vi "CRT Controller.vi"() -> ()   [LabVIEW 2016]
uses:
  HPTDC Driver Library Folder/Library files/Typedefs/TDCManager.ctl
  HPTDC Driver Library Folder/Library files/Typedefs/TDCHit.ctl
  VIs/Typedefs/Coincidence single histogram.ctl
  VIs/Typedefs/HitChart.ctl
  VIs/Typedefs/ROB display info.ctl
  <vilib>/addons/h5labview2/base/hid_t.ctl
  VIs/Typedefs/Hit chart cluster refnum.ctl
  <vilib>/Platform/TimedLoop/XDataNode/timing_clust.ctl
  <vilib>/Platform/TimedLoop/XDataNode/nitl_modes.ctl
  <vilib>/Platform/TimedLoop/XDataNode/wakeup.ctl
  HPTDC Driver Library Folder/Library files/Typedefs/TDCManagerRefnum.ctl
  VIs/Global Variables/Global AllowRead.vi
  VIs/Global Variables/AllowTDCHitsRead.vi
  VIs/Global Variables/AllowTDCFastRead.vi
  VIs/Global Variables/take CRT data.vi
  VIs/Global Variables/Master Ready For Data.vi
  VIs/Global Variables/Coincidence hunt limit.vi
  VIs/Global Variables/Program load indicators.vi
  VIs/Global Variables/AllowUserMessages.vi
  VIs/Global Variables/Coincidence Windows.vi
  VIs/Global Variables/System info.vi
  <vilib>/Instr/_visa.llb/VISA Configure Serial Port (Instr).vi
  <vilib>/platform/TimedLoop/XDataNode/XDataNode.xnode
  HPTDC Driver Library Folder/HPTDC Driver Library.lvlib
  <vilib>/Platform/TimedLoop/XDataNode/XDNodeRunTimeDep.lvlib
  <vilib>/addons/h5labview2/file/H5F.lvlib
  C:/Users/CRT Controller/CRTC Labview Application/Source/HPTDC Driver Library Folder/Library files/hptdc_net4_3.7.0_x64.dll
  HPTDC Driver Library Folder/Library files/hptdc_net4_3.7.0_x64.dll
panel:
  out "charactirzator refnum":refnum<vi>
  out "TDC Command Queue":string[](array[string])
  in  "Tab Control":T1(tab)
  in  "Hit rate save granularity in minutes":i32=1 min=1 step=1
  in  "GPS information save granularity in minutes":i32=1 min=1 step=1
  out "TDCRead":dbl(knob) scale=0.0..3300.0
  in  "Open coincrate":bool
  in  "Open trigrate":bool
  in  "Open EventDisplay":bool
  out "Run initiated at":timestamp
  out "Run ID":i32
  in  "Start Run":bool
  in  "ROB information save granularity in minutes":i32=15 min=1 step=1
  out "~Reads/s":u64
  in  "Planar coincidence window":i32=5 min=1 step=1 format="±%d ns"
  in  "Coincidence grouping window":i32=10 format="%d ns"
  out "Coincidences analysis overload":bool
  out "Coinchunt overflow":bool caption="Coincidence hunt overload"
  out "TDCRead overflow":bool caption="TDC readout overload"
  out "Sorter overflow":bool caption="Sorter overload"
  out "Coincidencehunt limit":dbl(knob) scale=0.0..900.0
  in  "Disable rail monitor":bool
  in  "Disable 15":bool
  in  "Enable 15":bool
  in  "Disable auto latch reset":bool
  in  "Verbosity":u8
  in  "Set Debug Verbosity":bool
  in  "Overvoltage":sgl=3.0 min=0 max=100 step=0.01 format="%#_4g V"
  in  "Set MPPCovervoltage":bool
  in  "Rep trigthres":bool
  in  "ROB hard reset":bool
  in  "disable amp":bool
  in  "Enable amp":bool caption="Enable"
  in  "Enable usermessages":bool=TRUE
  in  "Reset latch":bool
  in  "disable +-5V":bool
  in  "Enable +-5":bool
  in  "Disable 3.3":bool
  in  "Enable 3.3":bool
  in  "Voltage ref":u16(ring) items=["Default (internal)", "External"]
  in  "Continuous test charge":bool
  in  "Rep Temp":bool
  in  "Hard-set value":bool
  in  "VTrig mV":sgl min=0 max=1000 step=1 format="%#_2g mV"
  in  "Disable auto-VBias":bool
  in  "Bias voltage":sgl min=0 max=100 step=0.01 format="%#_4g V"
  in  "Set MPPC Bias":bool
  in  "VTrig percent":sgl min=0 max=100 step=0.1 format="%#_4g %"
  in  "Set VTrig":bool
  in  "Board selector":u16(ring) items=["0", "1", "2", "3", "4", "5", "6", "7", "8", "9", "10", "11", "12", "13", "14", "15", "All boards"]
  in  "go to standby":bool
  in  "Go to ready":bool
  in  "go to running":bool
  in  "Rep voltages":bool
  in  "Rep status":bool
  in  "Rep disclatch":bool
  in  "Remove MPPC":bool
  in  "Insert test charge":bool
  in  "Set voltage reference":bool
  in  "Echo":bool
  out "ROB Info cluster":T3={"ROB Info-display"={"ID:"=0, "State:"="UNKNOWN", "Voltages"=-1, "Temp:"=-1.0, "Latch count:"=-1, "VRef:"=enum."Unknown", "Trigthres:"=-1, "MPPC EN"=FALSE, "Test charge"=FALSE, "Responding"=FALSE, "Last update"=timestamp(0 s since 1904-01-01)}, "ROB Info-display 2"={"ID:"=1, "State:"="UNKNOWN", "Voltages"=-1, "Temp:"=-1.0, "Latch count:"=-1, "VRef:"=enum."Unknown", "Trigthres:"=-1, "MPPC EN"=FALSE, "Test charge"=FALSE, "Responding"=FALSE, "Last update"=timestamp(0 s since 1904-01-01)}, "ROB Info-display 3"={"ID:"=2, "State:"="UNKNOWN", "Voltages"=-1, "Temp:"=-1.0, "Latch count:"=-1, "VRef:"=enum."Unknown", "Trigthres:"=-1, "MPPC EN"=FALSE, "Test charge"=FALSE, "Responding"=FALSE, "Last update"=timestamp(0 s since 1904-01-01)}, "ROB Info-display 4"={"ID:"=3, "State:"="UNKNOWN", "Voltages"=-1, "Temp:"=-1.0, "Latch count:"=-1, "VRef:"=enum."Unknown", "Trigthres:"=-1, "MPPC EN"=FALSE, "Test charge"=FALSE, "Responding"=FALSE, "Last update"=timestamp(0 s since 1904-01-01)}, "ROB Info-display 5"={"ID:"=4, "State:"="UNKNOWN", "Voltages"=-1, "Temp:"=-1.0, "Latch count:"=-1, "VRef:"=enum."Unknown", "Trigthres:"=-1, "MPPC EN"=FALSE, "Test charge"=FALSE, "Responding"=FALSE, "Last update"=timestamp(0 s since 1904-01-01)}, "ROB Info-display 6"={"ID:"=5, "State:"="UNKNOWN", "Voltages"=-1, "Temp:"=-1.0, "Latch count:"=-1, "VRef:"=enum."Unknown", "Trigthres:"=-1, "MPPC EN"=FALSE, "Test charge"=FALSE, "Responding"=FALSE, "Last update"=timestamp(0 s since 1904-01-01)}, "ROB Info-display 7"={"ID:"=6, "State:"="UNKNOWN", "Voltages"=-1, "Temp:"=-1.0, "Latch count:"=-1, "VRef:"=enum."Unknown", "Trigthres:"=-1, "MPPC EN"=FALSE, "Test charge"=FALSE, "Responding"=FALSE, "Last update"=timestamp(0 s since 1904-01-01)}, "ROB Info-display 8"={"ID:"=7, "State:"="UNKNOWN", "Voltages"=-1, "Temp:"=-1.0, "Latch count:"=-1, "VRef:"=enum."Unknown", "Trigthres:"=-1, "MPPC EN"=FALSE, "Test charge"=FALSE, "Responding"=FALSE, "Last update"=timestamp(0 s since 1904-01-01)}, "ROB Info-display 9"={"ID:"=8, "State:"="UNKNOWN", "Voltages"=-1, "Temp:"=-1.0, "Latch count:"=-1, "VRef:"=enum."Unknown", "Trigthres:"=-1, "MPPC EN"=FALSE, "Test charge"=FALSE, "Responding"=FALSE, "Last update"=timestamp(0 s since 1904-01-01)}, "ROB Info-display 10"={"ID:"=9, "State:"="UNKNOWN", "Voltages"=-1, "Temp:"=-1.0, "Latch count:"=-1, "VRef:"=enum."Unknown", "Trigthres:"=-1, "MPPC EN"=FALSE, "Test charge"=FALSE, "Responding"=FALSE, "Last update"=timestamp(0 s since 1904-01-01)}, "ROB Info-display 11"={"ID:"=10, "State:"="UNKNOWN", "Voltages"=-1, "Temp:"=-1.0, "Latch count:"=-1, "VRef:"=enum."Unknown", "Trigthres:"=-1, "MPPC EN"=FALSE, "Test charge"=FALSE, "Responding"=FALSE, "Last update"=timestamp(0 s since 1904-01-01)}, "ROB Info-display 12"={"ID:"=11, "State:"="UNKNOWN", "Voltages"=-1, "Temp:"=-1.0, "Latch count:"=-1, "VRef:"=enum."Unknown", "Trigthres:"=-1, "MPPC EN"=FALSE, "Test charge"=FALSE, "Responding"=FALSE, "Last update"=timestamp(0 s since 1904-01-01)}, "ROB Info-display 13"={"ID:"=12, "State:"="UNKNOWN", "Voltages"=-1, "Temp:"=-1.0, "Latch count:"=-1, "VRef:"=enum."Unknown", "Trigthres:"=-1, "MPPC EN"=FALSE, "Test charge"=FALSE, "Responding"=FALSE, "Last update"=timestamp(0 s since 1904-01-01)}, "ROB Info-display 14"={"ID:"=13, "State:"="UNKNOWN", "Voltages"=-1, "Temp:"=-1.0, "Latch count:"=-1, "VRef:"=enum."Unknown", "Trigthres:"=-1, "MPPC EN"=FALSE, "Test charge"=FALSE, "Responding"=FALSE, "Last update"=timestamp(0 s since 1904-01-01)}, "ROB Info-display 15"={"ID:"=14, "State:"="UNKNOWN", "Voltages"=-1, "Temp:"=-1.0, "Latch count:"=-1, "VRef:"=enum."Unknown", "Trigthres:"=-1, "MPPC EN"=FALSE, "Test charge"=FALSE, "Responding"=FALSE, "Last update"=timestamp(0 s since 1904-01-01)}, "ROB Info-display 16"={"ID:"=15, "State:"="UNKNOWN", "Voltages"=-1, "Temp:"=-1.0, "Latch count:"=-1, "VRef:"=enum."Unknown", "Trigthres:"=-1, "MPPC EN"=FALSE, "Test charge"=FALSE, "Responding"=FALSE, "Last update"=timestamp(0 s since 1904-01-01)}} {"ROB Info-display 16"."Last update" format="%<%X>T"; "ROB Info-display 16"."Trigthres:" format="%.0fmV"; "ROB Info-display 16"."Temp:" format="%.2f C"; "ROB Info-display 15"."Last update" format="%<%X>T"; "ROB Info-display 15"."Trigthres:" format="%.0fmV"; "ROB Info-display 15"."Temp:" format="%.2f C"; "ROB Info-display 14"."Last update" format="%<%X>T"; "ROB Info-display 14"."Trigthres:" format="%.0fmV"; "ROB Info-display 14"."Temp:" format="%.2f C"; "ROB Info-display 13"."Last update" format="%<%X>T"; "ROB Info-display 13"."Trigthres:" format="%.0fmV"; "ROB Info-display 13"."Temp:" format="%.2f C"; "ROB Info-display 12"."Last update" format="%<%X>T"; "ROB Info-display 12"."Trigthres:" format="%.0fmV"; "ROB Info-display 12"."Temp:" format="%.2f C"; "ROB Info-display 11"."Last update" format="%<%X>T"; "ROB Info-display 11"."Trigthres:" format="%.0fmV"; "ROB Info-display 11"."Temp:" format="%.2f C"; "ROB Info-display 10"."Last update" format="%<%X>T"; "ROB Info-display 10"."Trigthres:" format="%.0fmV"; "ROB Info-display 10"."Temp:" format="%.2f C"; "ROB Info-display 9"."Last update" format="%<%X>T"; "ROB Info-display 9"."Trigthres:" format="%.0fmV"; "ROB Info-display 9"."Temp:" format="%.2f C"; "ROB Info-display 8"."Last update" format="%<%X>T"; "ROB Info-display 8"."Trigthres:" format="%.0fmV"; "ROB Info-display 8"."Temp:" format="%.2f C"; "ROB Info-display 7"."Last update" format="%<%X>T"; "ROB Info-display 7"."Trigthres:" format="%.0fmV"; "ROB Info-display 7"."Temp:" format="%.2f C"; "ROB Info-display 6"."Last update" format="%<%X>T"; "ROB Info-display 6"."Trigthres:" format="%.0fmV"; "ROB Info-display 6"."Temp:" format="%.2f C"; "ROB Info-display 5"."Last update" format="%<%X>T"; "ROB Info-display 5"."Trigthres:" format="%.0fmV"; "ROB Info-display 5"."Temp:" format="%.2f C"; "ROB Info-display 4"."Last update" format="%<%X>T"; "ROB Info-display 4"."Trigthres:" format="%.0fmV"; "ROB Info-display 4"."Temp:" format="%.2f C"; "ROB Info-display 3"."Last update" format="%<%X>T"; "ROB Info-display 3"."Trigthres:" format="%.0fmV"; "ROB Info-display 3"."Temp:" format="%.2f C"; "ROB Info-display 2"."Last update" format="%<%X>T"; "ROB Info-display 2"."Trigthres:" format="%.0fmV"; "ROB Info-display 2"."Temp:" format="%.2f C"; "ROB Info-display"."Last update" format="%<%X>T"; "ROB Info-display"."Trigthres:" format="%.0fmV"; "ROB Info-display"."Temp:" format="%.2f C"}
  in  "enable autoread":bool
  in  "enable rail monitor":bool
  in  "Fast read":bool caption="Only register amount of hits, \nnot time or channel. Supports reading \nout at the maximum TDC speed."
  out "Status":u16(ring) items=["Uninitialized", "Not configured", "Configured", "Running", "Paused", "Shutdown"]
  in  "Continue tdc":bool
  in  "Pause tdc":bool
  in  "Stop tdc":bool
  in  "Start tdc":bool
  in  "Read Cfg Again":bool
  in  "Reconfigure":bool
  in  "Read config string":bool
  in  "TDC Config string":string="FallingEnable 1"
  out "Set Parameter Names":string[](array[string])
  in  "Get set param names":bool
  in  "TDC Configuration filepath":string="C:\\Users\\CRT Controller\\CRTC Labview Application\\Source\\global.cfg"
  out "Init success":bool
  out "Histograms cluster":T5 {"Cluster 33"."S:" format="%_3f"; "Cluster 32"."S:" format="%_3f"; "Cluster 31"."S:" format="%_3f"; "Cluster 30"."S:" format="%_3f"; "Cluster 29"."S:" format="%_3f"; "Cluster 28"."S:" format="%_3f"; "Cluster 27"."S:" format="%_3f"; "Cluster 26"."S:" format="%_3f"; "Cluster 25"."S:" format="%_3f"; "Cluster 24"."S:" format="%_3f"; "Cluster 23"."S:" format="%_3f"; "Cluster 22"."S:" format="%_3f"; "Cluster 21"."S:" format="%_3f"; "Cluster 20"."S:" format="%_3f"; "Cluster 19"."S:" format="%_3f"; "Cluster 18"."S:" format="%_3f"; "Cluster 17"."S:" format="%_3f"; "Cluster 16"."S:" format="%_3f"; "Cluster 15"."S:" format="%_3f"; "Cluster 14"."S:" format="%_3f"; "Cluster 13"."S:" format="%_3f"; "Cluster 12"."S:" format="%_3f"; "Cluster 11"."S:" format="%_3f"; "Cluster 10"."S:" format="%_3f"; "Cluster 9"."S:" format="%_3f"; "Cluster 8"."S:" format="%_3f"; "Cluster 7"."S:" format="%_3f"; "Cluster 6"."S:" format="%_3f"; "Cluster 5"."S:" format="%_3f"; "Cluster 4"."S:" format="%_3f"; "Cluster 3"."S:" format="%_3f"; "Cluster 2"."S:" format="%_3f"}
  in  "Histogram select":T6(ring)
  in  "MaxHistItems":i32=1000 caption="Number of elements"
  in  "SetMaxHistItems":bool
  in  "charts tab":enum32{"Top layer", "Bottom layer"}(tab)
  out "Top layer hit charts":T8 {"Waveform Chart 8"."ID" format="ch %d"; "Waveform Chart 7"."ID" format="ch %d"; "Waveform Chart 6"."ID" format="ch %d"; "Waveform Chart 5"."ID" format="ch %d"; "Waveform Chart 4"."ID" format="ch %d"; "Waveform Chart 3"."ID" format="ch %d"; "Waveform Chart 2"."ID" format="ch %d"; "Waveform Chart"."ID" format="ch %d"}
  out "Bottom layer hit charts":T8 {"Waveform Chart 8"."ID" format="ch %d"; "Waveform Chart 7"."ID" format="ch %d"; "Waveform Chart 6"."ID" format="ch %d"; "Waveform Chart 5"."ID" format="ch %d"; "Waveform Chart 4"."ID" format="ch %d"; "Waveform Chart 3"."ID" format="ch %d"; "Waveform Chart 2"."ID" format="ch %d"; "Waveform Chart"."ID" format="ch %d"}
  in  "Resolution(seconds)":dbl=5.0 min=0.1 step=1.0
  in  "Set chart res":bool
  in  "Clear charts":bool
  out "Coinc stats time":i32 caption="Seconds of coincidence statistics:"
  out "Coinc stats table":string[][](table) caption="Statistics of the latest coincidences"
  in  "GPS CMD Send Button":bool
  in  "GPS command input":string
  in  "Baud rate GPS":u32=38400 caption="Baud rate"
  in  "GPS serial port":refnum<visa-resource-name>="COM7"
  in  "Open GPS Port":bool caption="Open ROB Port"
  in  "Open Master Port":bool
  in  "Baud rate sniffer":u32=9600 caption="Baud rate"
  in  "Sniffer serial port":refnum<visa-resource-name>
  in  "Open Sniffer Port":bool
  in  "Baud rate ROB":u32=9600 caption="Baud rate"
  in  "ROB serial port":refnum<visa-resource-name>
  in  "Open ROB Port":bool
  in  "Baud rate master":u32=115200 caption="Baud rate"
  in  "Master serial port":refnum<visa-resource-name>="COM3"
  out "Master Serial Input Data":string
  out "Sniffer Serial Input Data":string
  out "ROB Serial Input Data":string
  out "GPS serial input data":string
  out "Initiate finished":bool
  out "Programmatic set trigthres":bool
  in  "Data recording root path":path=path "D:/Data/2018"
  in  "run counter path":path=path "C:/Users/CRT Controller/CRTC Labview Application/Source/Configurations etc/Run counter.txt"
  out "Programmatic rep disclatch":bool
  out "Programmatic rep temp":bool
  out "Programmatic rep stat":bool
  out "Programmatic rep volts":bool
  out "Command Queue":string[](array[string])
  out "StopNotifier":refnum<notifier>
  out "Sniffer serial port":refnum<visa-resource-name>
  out "ROB serial port":refnum<visa-resource-name>
  out "Master serial port":refnum<visa-resource-name>
  out "TDCHitsQueue":refnum<queue>
  in  "TDCManager":T9
  out "Master data":u8[][](array[numeric])
  out "Sorter Refnum":refnum<vi>
  out "TDCRead Refnum":refnum<vi>
  out "TDCFastRead Refnum":refnum<vi>
  out "MasterSerial Refnum":refnum<vi>
  out "SnifferSerial Refnum":refnum<vi>
  out "ROBSerial Refnum":refnum<vi>
  out "Daily datafile reference":T10 format="%.0x"
  out "Master command sender refnum":refnum<vi>
  out "Added time":u64
  out "Coinchunt Lim":i32
  out "MasterCmdQueue":refnum<queue>
  out "error out":errorcluster
  out "TDCStart time":timestamp
  out "Event display Refnum":refnum<vi>
  out "Current day":i32
  out "Trig chara refnum":refnum<vi>
  out "GPS serial port":refnum<visa-resource-name>
  out "GPSSerial Refnum":refnum<vi>
  out "GpsDataQueue":refnum<queue>
  out "hit charts refnum cluster":T12
  in  "stop":bool
  # "Debug things. No need to touch this in normal operation..."
  # "Rail monitor"
  # "15V"
  # "3.3V"
  # "+-5V"
  # "Amplifier"
  # "This table shows the total amount of registered coincidences over the last 10000 seconds or so. The top coloumns indicates that, for a block of coincidences, how many were present in the top plane. The rows indicate how many were present in the bottom plane. \nSo if 1x1 has the highest number, that means it is most common for a single coincidence on the top plane and a single coincidence on the bottom plane to occur simulatenously (within the CRT-wide coincidence window).\nIt is unlikely that more than a few coincidences will occur simulatenously, but up to 10x10 has been added to the table to spot unforeseen problems."
  # "These items are internal variables used by the CRTC and \ncannot be modified or should not be modified."
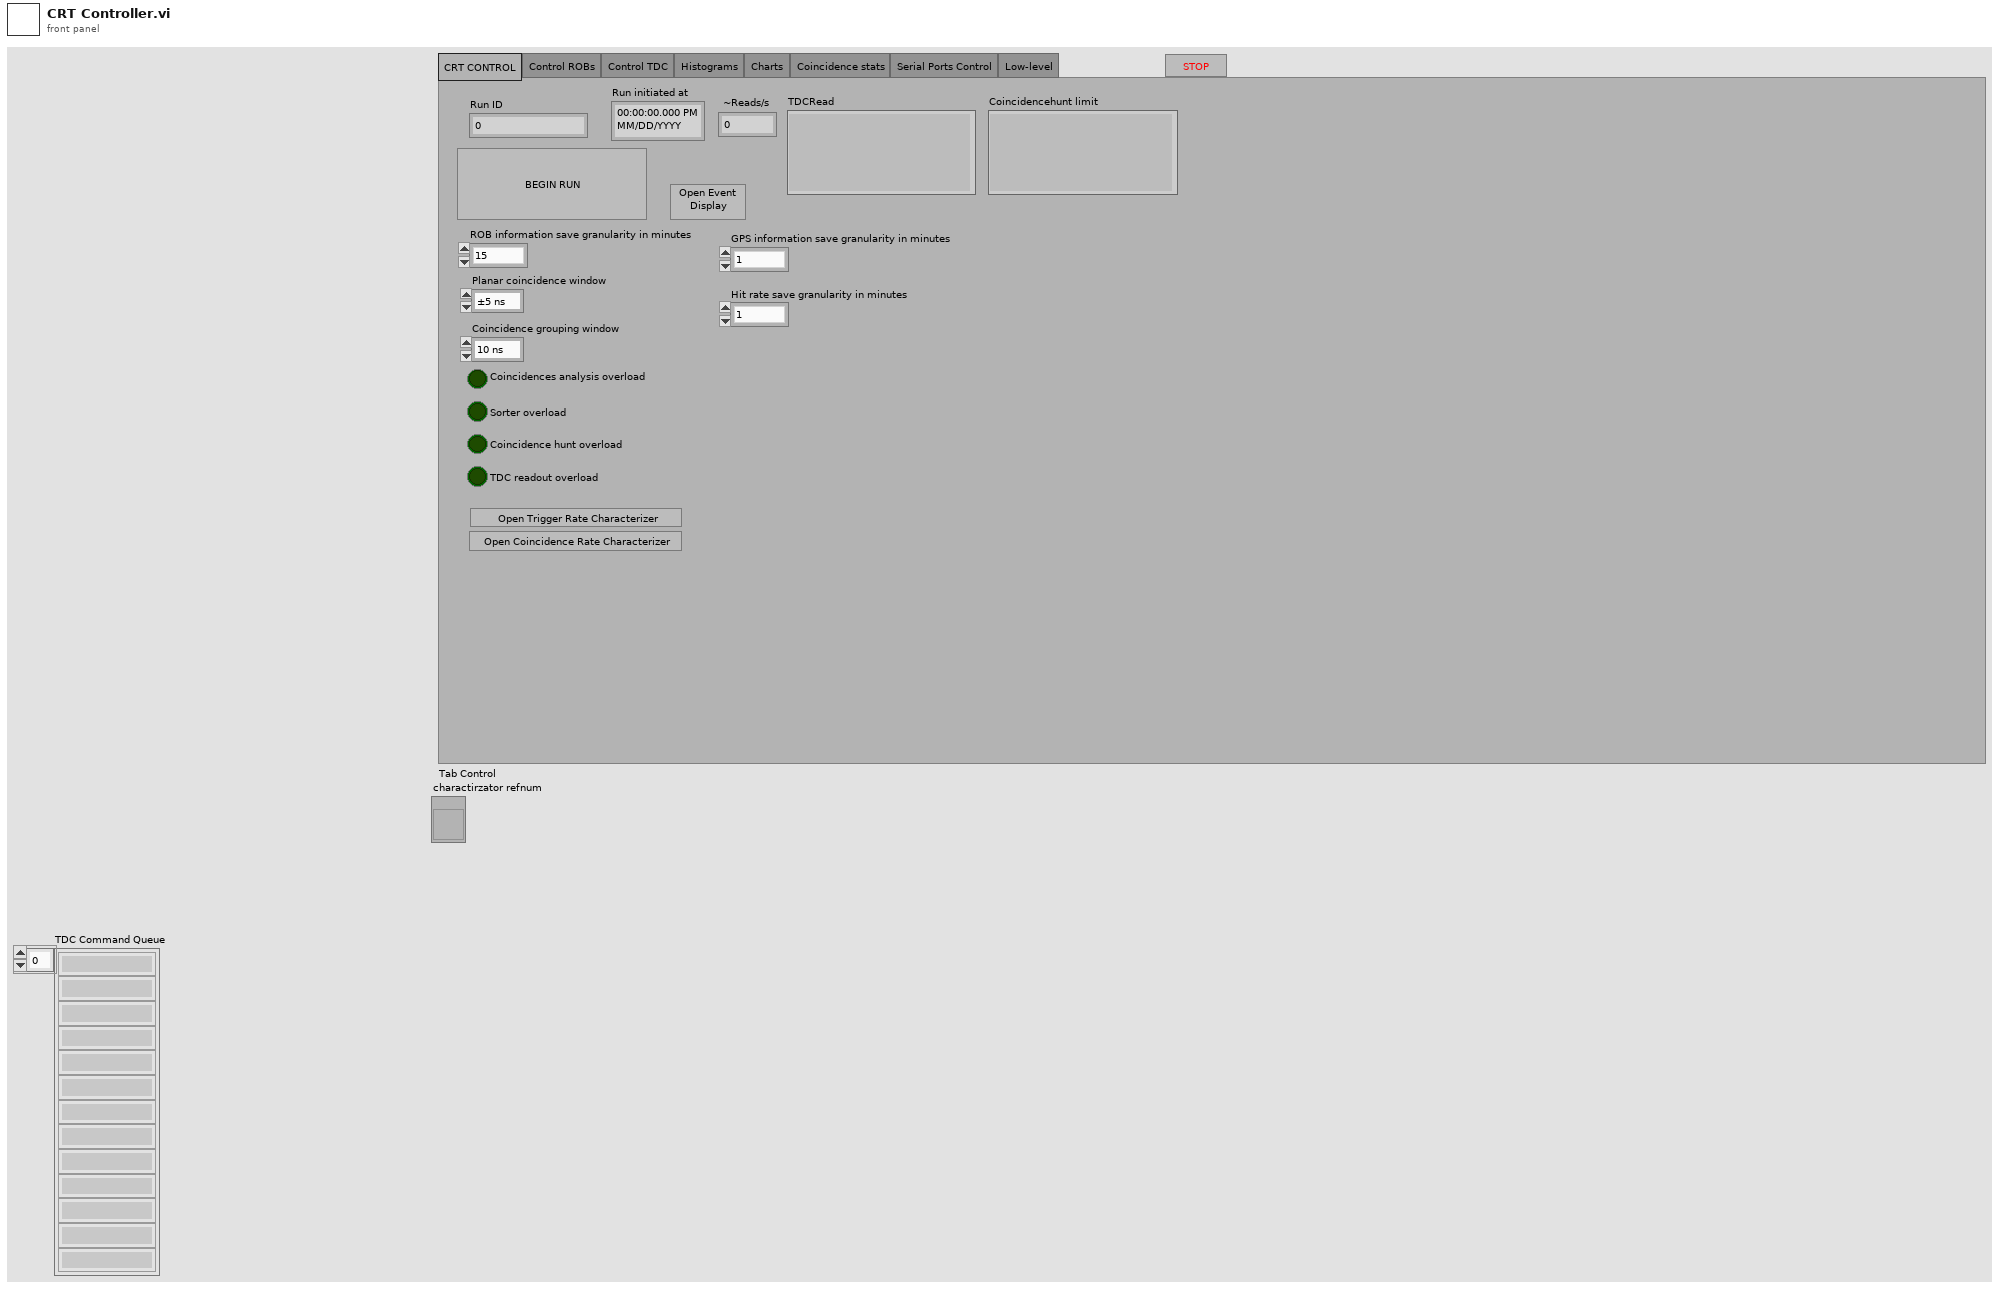
[diagram p1: front panel]
types:
  T1 = enum32{"CRT CONTROL", "Control ROBs", "Control TDC", "Histograms", "Charts", "Coincidence stats", "Serial Ports Control", "Low-level"}
  T2 = typedef "ROB display info.ctl" = cluster{"ID:":i32, "State:":string, "Voltages":i32, "Temp:":dbl, "Latch count:":i32, "VRef:":enum16{"External", "Internal", "Unknown"}, "Trigthres:":i32, "MPPC EN":bool, "Test charge":bool, "Responding":bool, "Last update":timestamp}
  T3 = cluster{"ROB Info-display":T2, "ROB Info-display 2":T2, "ROB Info-display 3":T2, "ROB Info-display 4":T2, "ROB Info-display 5":T2, "ROB Info-display 6":T2, "ROB Info-display 7":T2, "ROB Info-display 8":T2, "ROB Info-display 9":T2, "ROB Info-display 10":T2, "ROB Info-display 11":T2, "ROB Info-display 12":T2, "ROB Info-display 13":T2, "ROB Info-display 14":T2, "ROB Info-display 15":T2, "ROB Info-display 16":T2}
  T4 = typedef "Coincidence single histogram.ctl" = cluster{"Histogram Graph":cluster{"X Values":dbl[], "Histogram: h(x)":i32[]}[], "IDs":i8[], "Datapoints:":i32, "S:":dbl, "Data array":cluster{"Data":i32[], "Max index":i32, "Current index":i32, "Numofpoints":i32}}
  T5 = cluster{"Cluster 2":T4, "Cluster 3":T4, "Cluster 4":T4, "Cluster 5":T4, "Cluster 6":T4, "Cluster 7":T4, "Cluster 8":T4, "Cluster 9":T4, "Cluster 10":T4, "Cluster 11":T4, "Cluster 12":T4, "Cluster 13":T4, "Cluster 14":T4, "Cluster 15":T4, "Cluster 16":T4, "Cluster 17":T4, "Cluster 18":T4, "Cluster 19":T4, "Cluster 20":T4, "Cluster 21":T4, "Cluster 22":T4, "Cluster 23":T4, "Cluster 24":T4, "Cluster 25":T4, "Cluster 26":T4, "Cluster 27":T4, "Cluster 28":T4, "Cluster 29":T4, "Cluster 30":T4, "Cluster 31":T4, "Cluster 32":T4, "Cluster 33":T4}
  T6 = enum16{"All histograms", "0x4", "0x5", "0x6", "0x7", "1x4", "1x5", "1x6", "1x7", "2x4", "2x5", "2x6", "2x7", "3x4", "3x5", "3x6", "3x7", "8x12", "8x13", "8x14", "8x15", "9x12", "9x13", "9x14", "9x15", "10x12", "10x13", "10x14", "10x15", "11x12", "11x13", "11x14", "11x15"}
  T7 = typedef "HitChart.ctl" = cluster{"Waveform Chart":cluster{"Coincidences":dbl, "Non-coincidences":dbl, "Ratio":dbl, "Total hits":dbl}[], "Last update timestamp":timestamp, "Resolution(s)":dbl, "nondisplayed coincs":i32, "nondisplayed noncoincs":i32, "Last upd":i64, "ID":i8}
  T8 = cluster{"Waveform Chart":T7, "Waveform Chart 2":T7, "Waveform Chart 3":T7, "Waveform Chart 4":T7, "Waveform Chart 5":T7, "Waveform Chart 6":T7, "Waveform Chart 7":T7, "Waveform Chart 8":T7}
  T9 = typedef "HPTDC Driver Library.lvlib/TDCManager.ctl" = refnum<k24>
  T10 = typedef "hid_t.ctl" = i32
  T11 = typedef "Hit chart cluster refnum.ctl" = refnum<vi>
  T12 = cluster{"Hit charts top":T11, "Hit charts bottom":T11}
  T13 = cluster{"Data":string, "Port":refnum<visa-resource-name>}
  T14 = typedef "HPTDC Driver Library.lvlib/TDCHit.ctl" = cluster{"channel":u8, "time":u64, "type":u8}
  T15 = typedef "XDNodeRunTimeDep.lvlib/timing_clust.ctl" = cluster{"Expected End [f-1]":u64, "Actual End [f-1]":u64, "Finished Late? [f-1]":bool, "Expected End [i-1]":u64, "Actual End [i-1]":u64, "Finished Late? [i-1]":bool, "Expected Start [i]":u64, "Actual Start [i]":u64, "Expected Start [f]":u64, "Actual Start [f]":u64, "Source Name":string, "Structure Name":string, "Period":i64, "Deadline":i64, "Offset":i64, "Start":i64, "Priority":i32, "Timeout":i32, "Mode":T16, "Wakeup Reason":T17, "Error":errorcluster, "Source Type":string, "Secondary Source Type":string, "Global End Time":u64, "Global Start Time":u64, "Frame Duration":u64, "Iteration Duration":u64, "Assigned CPU":i32, "I/O Scan Engine Mode":u32}
  T16 = typedef "XDNodeRunTimeDep.lvlib/nitl_modes.ctl" = enum32{"No Change", "Process missed periods, maintain original phase", "Discard missed periods, maintain original phase", "Process missed periods, ignore original phase", "Discard missed periods, ignore original phase"}
  T17 = typedef "XDNodeRunTimeDep.lvlib/wakeup.ctl" = enum32{"Normal", "Aborted", "Asynchronous wakeup", "Timing source error", "Timed loop error", "Timeout"}
  T18 = enum16{"Reset", "ReadAndReset", "Read", "Add", "Init"}
  T19 = enum16{"big-endian, network order", "native, host order", "little-endian"}
  T20 = enum8{"Enabled", "Disabled", "Disabled and Grayed Out"}
  T21 = enum32{"Invalid", "Standard", "Closed", "Hidden", "Minimized", "Maximized"}
  T22 = cluster{"VTrig mV":refnum<vi>, "Top hit charts":T11, "Bottom hit charts":T11, "Board selector":refnum<vi>, "VTrig percent ":refnum<vi>, "Hard-set value":refnum<vi>, "Programmatic set trigthres":refnum<vi>}
  T23 = enum16{"insertPPS", "insertUTC", "read", "initiate"}
  T24 = cluster{"VISAResourceName in":refnum<vi>, "Input buffer refnum":refnum<vi>}
  T25 = cluster{"Master data ref":refnum<vi>, "VISAResourceName in":refnum<vi>, "Input buffer refnum":refnum<vi>}
  T26 = typedef "TDCManagerRefnum.ctl" = refnum<vi>
  T27 = cluster{"TDCManager Refnum":T26, "Unable to keep up indicator":refnum<vi>}
  T28 = cluster{"TDCManager Refnum":T26, "Queue overflow indicator":refnum<vi>, "Hit rate warning":refnum<vi>}
  T29 = typedef "Semaphore RefNum" = refnum<k1>
  T30 = cluster{"Hit charts bottom":T11, "Hit charts top":T11, "Hitrate save granularity in minutes":refnum<vi>}
  T31 = enum16{"Null", "BottomLayer", "TopAndBottom", "TopLayer"}
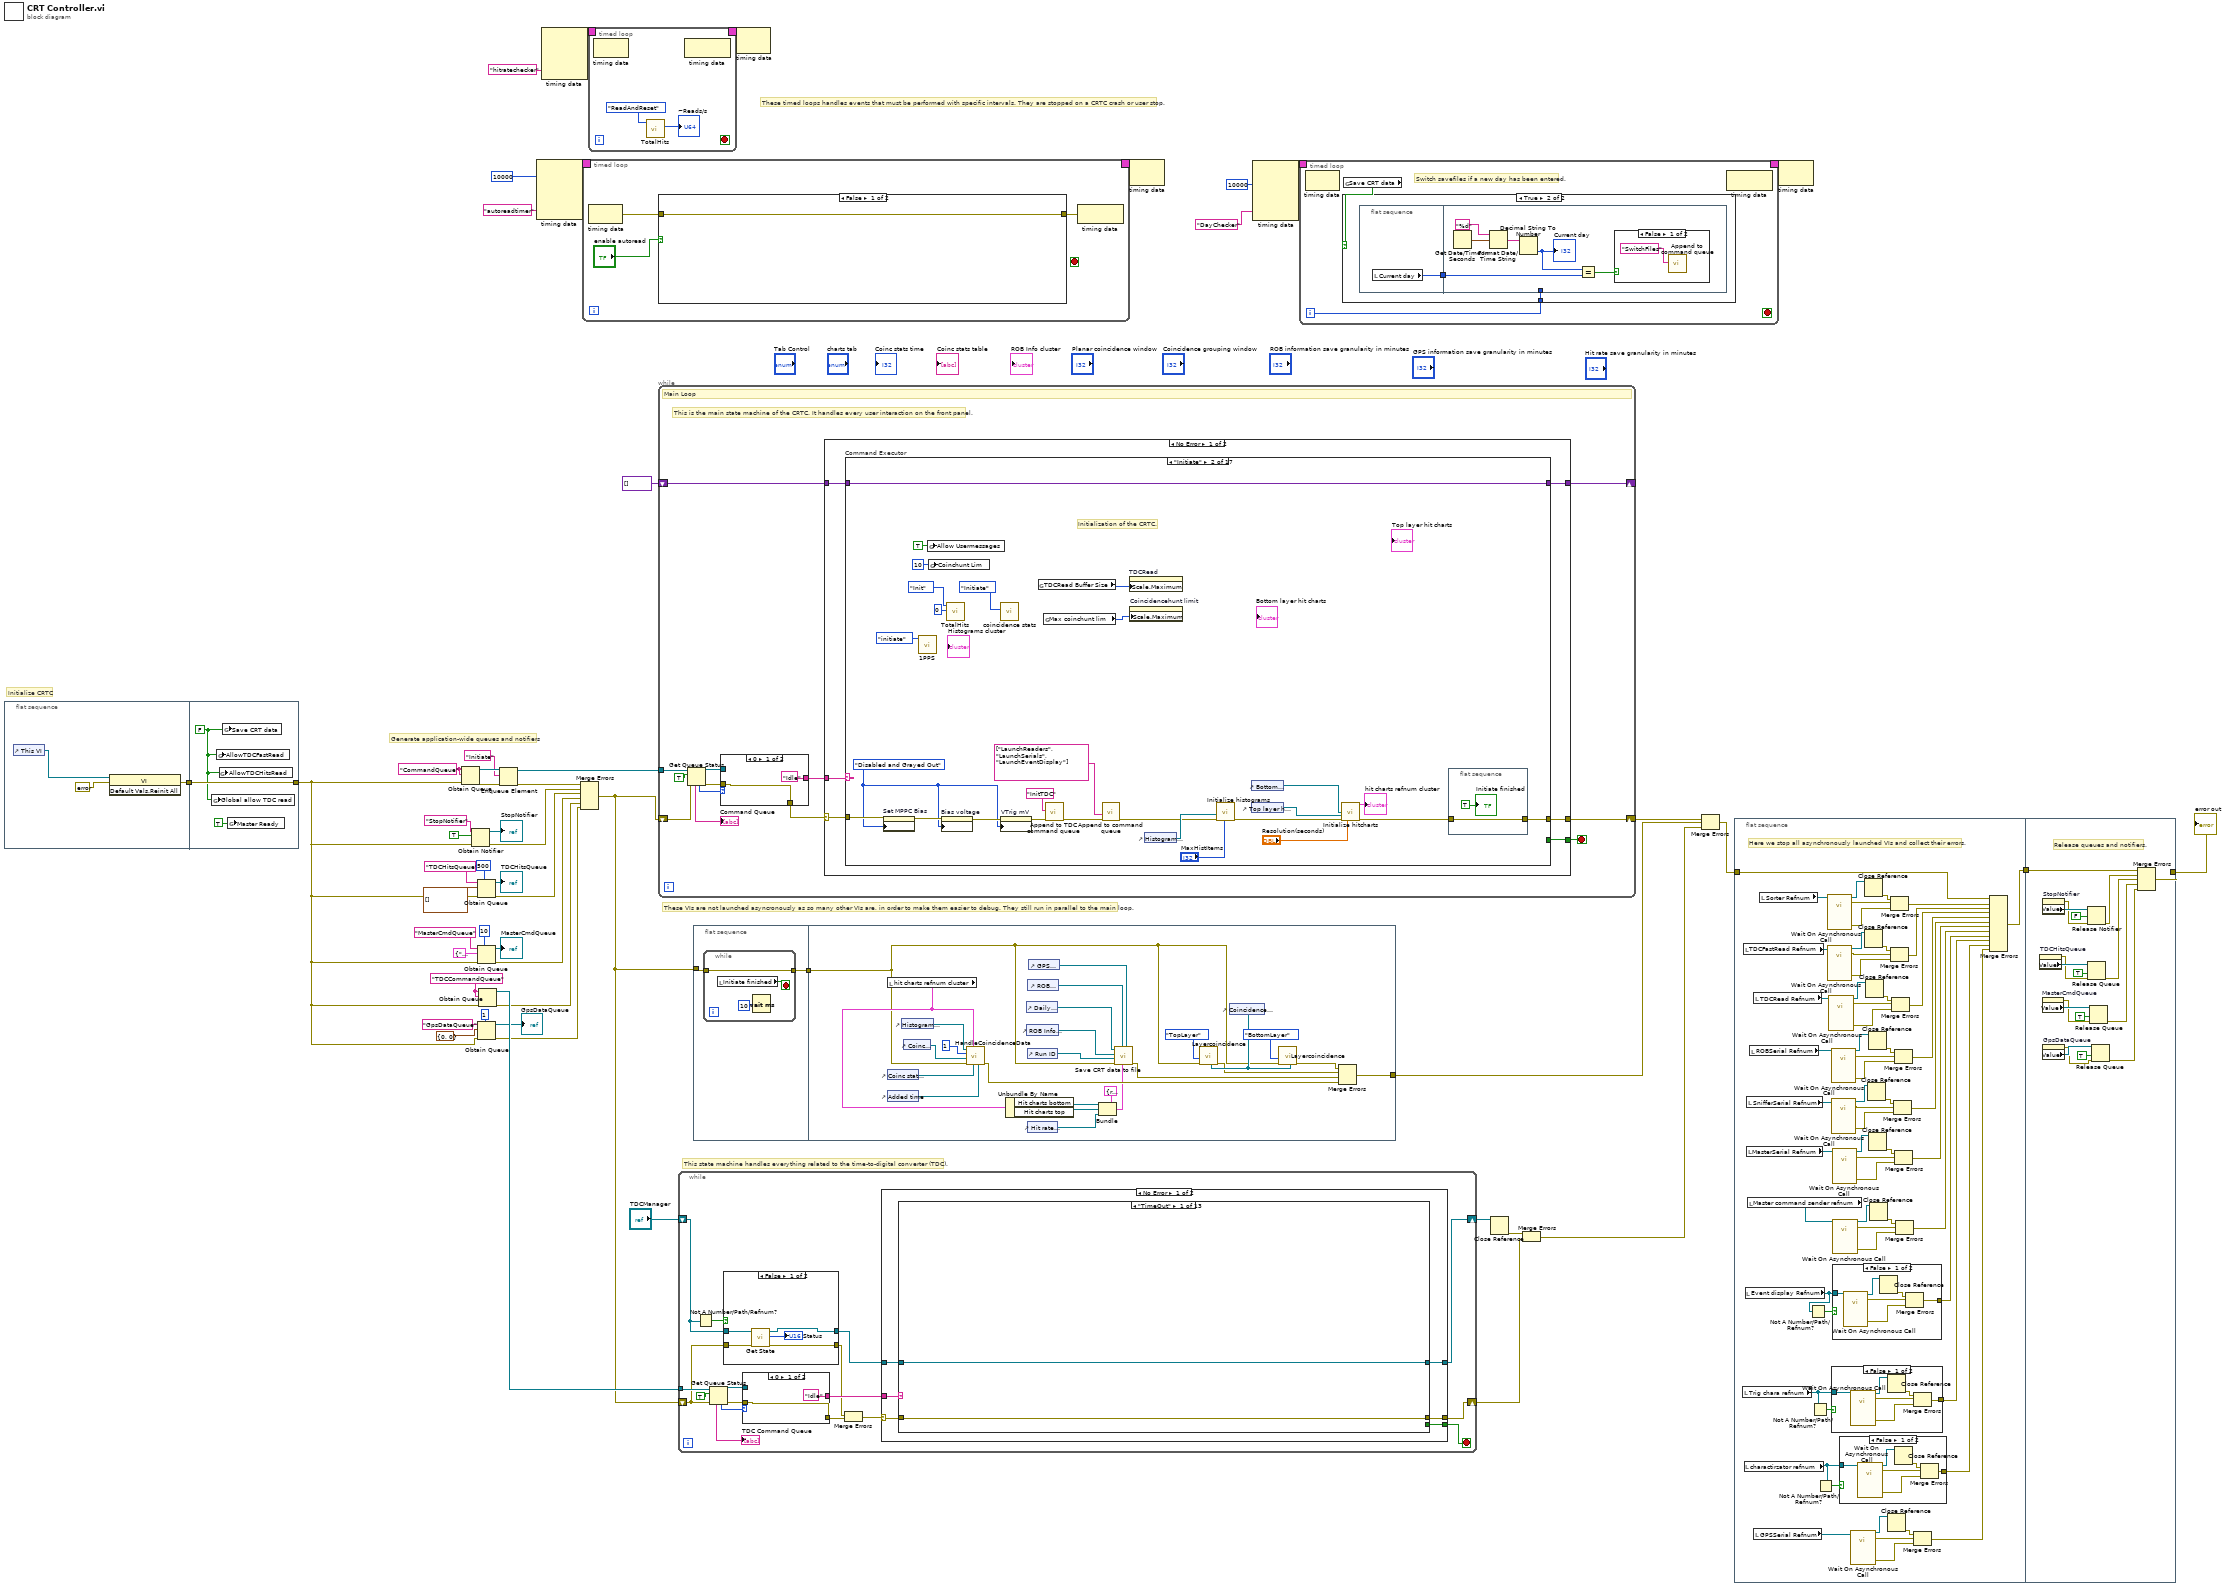
[diagram p0: block diagram]
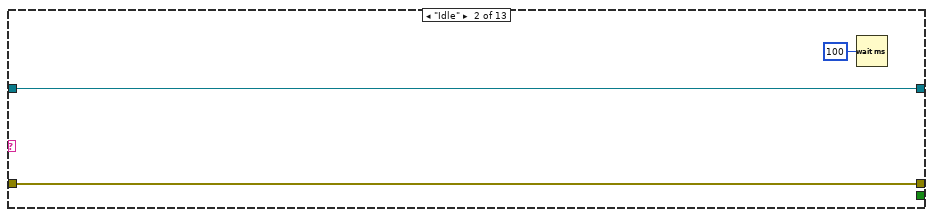
[diagram p3: hidden frame]
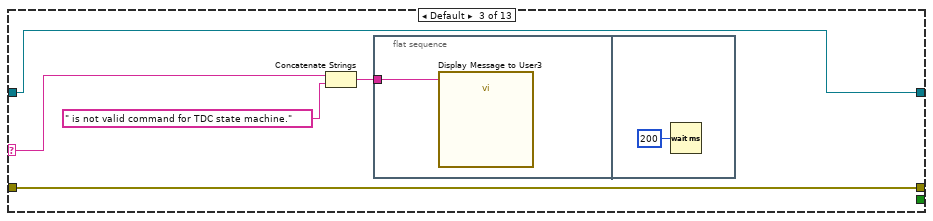
[diagram p4: hidden frame]
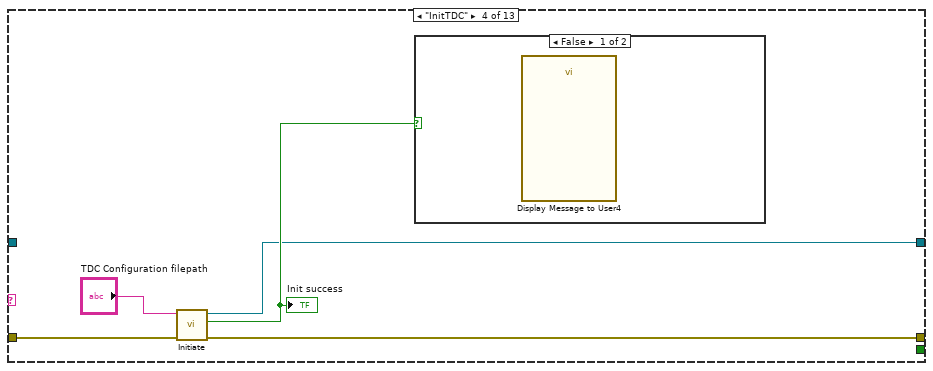
[diagram p5: hidden frame]
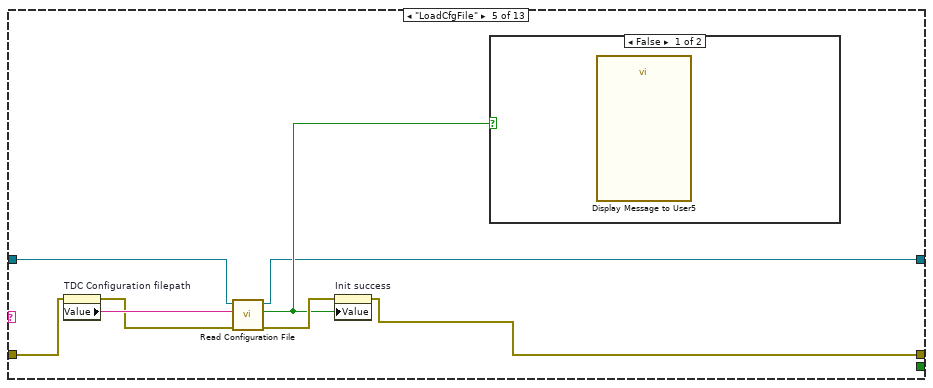
[diagram p7: hidden frame]
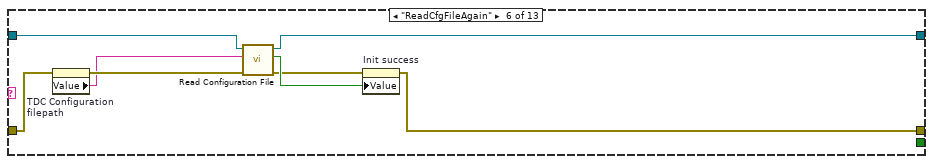
[diagram p9: hidden frame]
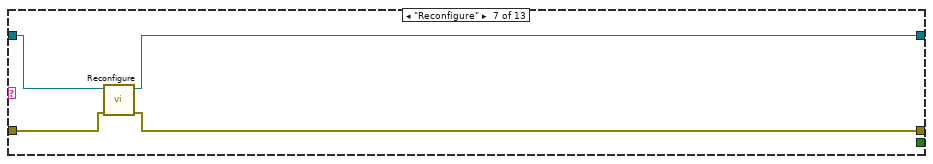
[diagram p10: hidden frame]
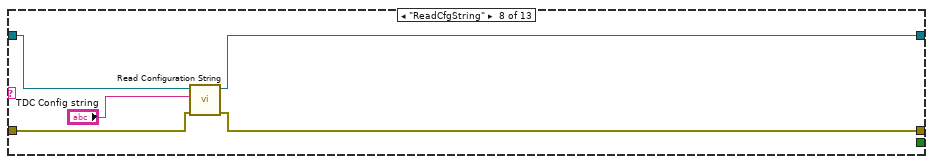
[diagram p11: hidden frame]
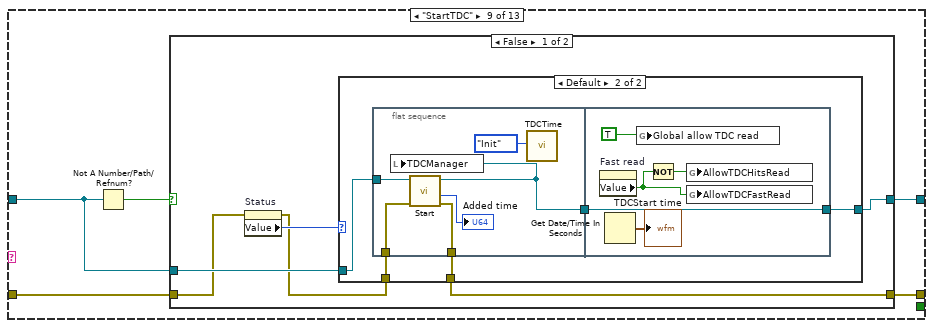
[diagram p12: hidden frame]
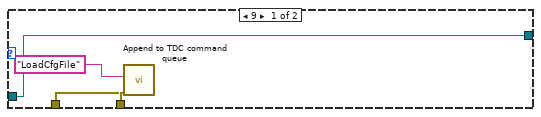
[diagram p13: hidden frame]
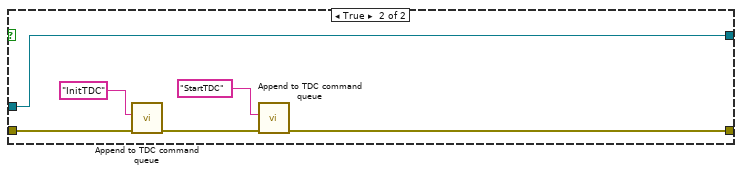
[diagram p14: hidden frame]
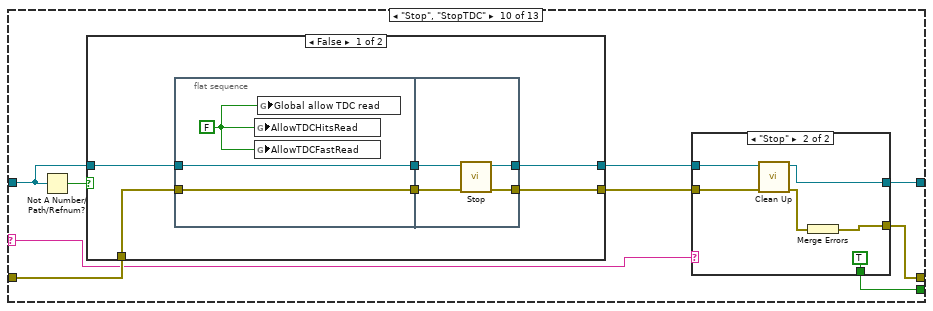
[diagram p15: hidden frame]
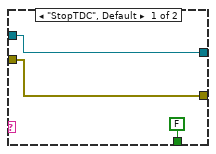
[diagram p16: hidden frame]
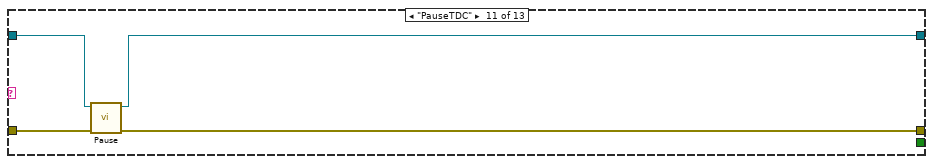
[diagram p18: hidden frame]
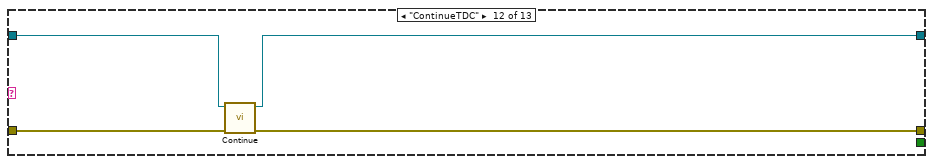
[diagram p19: hidden frame]
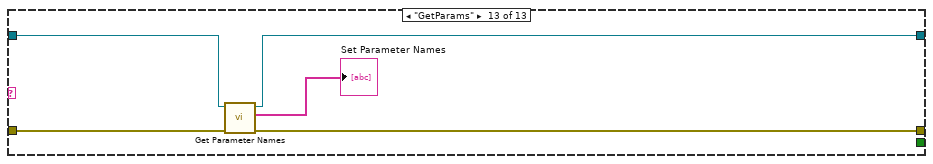
[diagram p20: hidden frame]
diagram:
  w40 = "TDCCommandQueue" ("name (unnamed)")
  w54 = "CommandQueue" ("name (unnamed)")
  # "This state machine handles everything related to the time-to-digital converter (TDC)."
  # "These VIs are not launched asyncronously as so many other VIs are, in order to make them easier to debug. They still run in parallel to the main loop."
  # "These timed loops handles events that must be performed with specific intervals. They are stopped on a CRTC crash or user stop."
  # "Generate application-wide queues and notifiers"
  # "Initialize CRTC"
  n1 = flat-sequence {
    tunnel: [w56] -> w33
    tunnel: [w60] -> w6
    tunnel: w33 -> [w60]
    frame #0 {
      n2 = control-ref of="This VI"() -> (w57:refnum<vi>)
      n3 = invoke class="VI" method="Default Vals.Reinit All"(reference=w57, error in=errorcluster {"status"=FALSE, "code"=0, "source"=""} ("error in (no error)")) -> (error out=w56:errorcluster)  [unwired: 1 in, 2 out]
    }
    frame #1 {
      w59 = FALSE ("Save CRT data")
      n4 = global write "Global AllowRead.vi" "Global allow TDC read"(w59) -> ()
      n5 = global write "AllowTDCFastRead.vi" "AllowTDCFastRead"(w59) -> ()
      n6 = global write "AllowTDCHitsRead.vi" "AllowTDCHitsRead"(w59) -> ()
      n7 = global write "take CRT data.vi" "Save CRT data"(w59) -> ()
      n8 = global write "Master Ready For Data.vi" "Master Ready"(TRUE ("Master Ready")) -> ()
    }
  }
  n9 = Obtain Queue(name (unnamed)=w54, element data type=w54, error in (no error)=w6) -> (queue out=w52:refnum<queue>, error out=w50:errorcluster)  [unwired: 2 in, 1 out]
  n10 = Obtain Notifier(name (unnamed)="StopNotifier", notification data type=TRUE, error in (no error)=w6) -> (notifier out=→"StopNotifier":refnum<notifier>, error out=w44:errorcluster)  [unwired: 1 in, 1 out]
  n11 = Obtain Queue(max queue size (-1, unlimited)=500, name (unnamed)="TDCHitsQueue", element data type=T14[] [] ("TDCHits"), error in (no error)=w6) -> (queue out=→"TDCHitsQueue":refnum<queue>, error out=w15:errorcluster)  [unwired: 1 in, 1 out]
  n12 = Obtain Queue(max queue size (-1, unlimited)=10, name (unnamed)="MasterCmdQueue", element data type=T13 {"Data"="", "Port"=""} ("Cluster"), error in (no error)=w6) -> (queue out=→"MasterCmdQueue":refnum<queue>, error out=w14:errorcluster)  [unwired: 1 in, 1 out]
  n13 = Obtain Queue(max queue size (-1, unlimited)=1, name (unnamed)="GpsDataQueue", element data type=cluster{"Fix quality":i8, "Satelites":i8} {"Fix quality"=0, "Satelites"=0}, error in (no error)=w6) -> (queue out=→"GpsDataQueue":refnum<queue>, error out=w5:errorcluster)  [unwired: 1 in, 1 out]
  n14 = Obtain Queue(name (unnamed)=w40, element data type=w40, error in (no error)=w6) -> (queue out=w39:refnum<queue>, error out=w13:errorcluster)  [unwired: 2 in, 1 out]
  n15 = Enqueue Element(queue=w52, element="Initiate", error in (no error)=w50) -> (queue out=w53:refnum<queue>, error out=w45:errorcluster)  [unwired: 1 in, 1 out]
  n16 = node-c288(i64 10000 ("Period"), "autoreadtimer" ("Structure Name")) -> (w31:T15)  [unwired: 3 in]
  n17 = node-c288("hitratechecker" ("Structure Name")) -> (w19:T15)  [unwired: 3 in]
  n18 = Merge Errors(w45, w44, w15, w14, w13, w5) -> (w2:errorcluster)
  n19 = timed-loop {
    timing: w31 -> [_]
    timing-out: [_] -> w30
    stop <- _ stop-if-true
    n20 = node-c288() -> (w63:errorcluster)  [unwired: 1 in]
    n21 = case shown="False" "enable autoread" {
      tunnel: w63 -> [w64 w68]
      tunnel: [w64 w65] -> w62
      frame False {
      }
      frame True {
        w66 = TRUE
        n22 = property on="Programmatic rep volts" class="Bool (strict)"(error in=w68, "Val(Sgnl)"=w66) -> (error out=w69:errorcluster)  [unwired: 1 in, 1 out]
        n23 = property on="Programmatic rep temp" class="Bool (strict)"(error in=w69, "Val(Sgnl)"=w66) -> (error out=w67:errorcluster)  [unwired: 1 in, 1 out]
        n24 = property on="Programmatic rep stat" class="Bool (strict)"(error in=w67, "Val(Sgnl)"=w66) -> (error out=w70:errorcluster)  [unwired: 1 in, 1 out]
        n25 = property on="Programmatic rep disclatch" class="Bool (strict)"(error in=w70, "Val(Sgnl)"=w66) -> (error out=w65:errorcluster)  [unwired: 1 in, 1 out]
      }
    }
    n26 = node-c288(w62) -> ()  [unwired: 1 out]
  }
  n27 = timed-loop {
    timing: w19 -> [_]
    timing-out: [_] -> w18
    stop <- _ stop-if-true
    n28 = node-c288() -> ()  [unwired: 1 in, 1 out]
    n29 = call "TotalHits.vi"("Action"=T18."ReadAndReset") -> ("Result"=→"~Reads/s":u64)  [unwired: 10 in]
    n30 = node-c288() -> ()  [unwired: 1 in, 1 out]
  }
  n31 = while {
    tunnel: w53 -> [w88]
    shift-right: [w84] -> w48
    shift-left: w2 -> [w85]
    shift-right: [w81] -> _
    shift-left: variant[] [] -> [w82]
    stop <- w83 stop-if-true
    # "This is the main state machine of the CRTC. It handles every user interaction on the front panel."
    # "Main Loop"
    n32 = Get Queue Status(queue=w88, return elements? (F)=TRUE, error in (no error)=w85) -> (queue out=w91:refnum<queue>, error out=w90:errorcluster, # elements in queue=w92:i32, elements=→"Command Queue":string[])  [unwired: 4 out]
    n33 = case shown="0" w92 {
      tunnel: ["Idle" ("element") w1258] -> w86
      tunnel: w91 -> [_ w1264]
      tunnel: w90 -> [w1254 w1263]
      tunnel: [w1254 w1257] -> w80
      frame 0 {
      }
      frame Default {
        n34 = Dequeue Element(queue=w1264, timeout in ms (-1)=50, error in (no error)=w1263) -> (element=w1262:string, timed out?=w1261:bool, error out=w1257:errorcluster)  [unwired: 1 out]
        n35 = Not(x=w1261) -> (.not. x?=w1260:bool)
        n36 = Select(t=w1262, s=w1260, f="TimeOut") -> (s? t:f=w1258:string)
      }
    }
    n37 = case shown="No Error" w80 {
      selector: w80 -> [w93 w1218]
      tunnel: w86 -> [w98 _]
      tunnel: [w97 w1221] -> w84
      tunnel: [w96 TRUE] -> w83
      tunnel: w82 -> [w95 w1252]
      tunnel: [w94 w1252] -> w81
      frame No Error {
        n38 = case "Command Executor" shown="\"Initiate\"" w98 {
          selector: w98 -> [_ _ _ _ _ _ _ w959 _ _ _ _ _ _ _ _ _]
          tunnel: [w104 w829 w864 w900 w911 w915 w923 w958 w974 w999 w1010 w1074 w1108 w1134 w1157 w1173 w1210] -> w97
          tunnel: w93 -> [w105 w853 w874 w901 w910 w915 w950 w958 w976 w1006 w1020 w1081 w1112 w1135 w1158 w1177 w1211]
          tunnel: [_ _ _ _ _ _ TRUE _ _ _ _ _ _ _ _ _ _] -> w96
          tunnel: w95 -> [w103 w854 w862 w899 w902 w914 w955 w957 w988 w1009 w1027 w1073 w1107 w1133 w1156 w1172 w1208]
          tunnel: [w102 w854 w862 w899 w902 w914 w955 w957 _ _ _ w1073 w1107 w1133 w1156 w1172 w1208] -> w94
          frame "Idle" {
            n39 = global read "Program load indicators.vi" "Coincidence hunt limit"() -> (→"Coincidencehunt limit":i32)
            n40 = global read "Program load indicators.vi" "Reads per TDC call"() -> (→"TDCRead":i32)
            n41 = global read "Coincidence hunt limit.vi" "Coinchunt Lim"() -> (→"Coinchunt Lim":i32)
            n42 = event shown="[48] \"Open coincrate\": Value Change" {
              selector: _ -> [_ _ _ _ _ _ _ _ _ _ _ _ _ _ _ _ _ _ _ _ _ _ _ _ _ _ _ _ _ _ _ _ _ _ _ _ _ _ _ _ _ _ _ _ _ _ _ _ _]
              dyn-events: _ -> [_ _ _ _ _ _ _ _ _ _ _ _ _ _ _ _ _ _ _ _ _ _ _ _ _ _ _ _ _ _ _ _ _ _ _ _ _ _ _ _ _ _ _ _ _ _ _ _ _]
              timeout: 100 -> [_ _ _ _ _ _ _ _ _ _ _ _ _ _ _ _ _ _ _ _ _ _ _ _ _ _ _ _ _ _ _ _ _ _ _ _ _ _ _ _ _ _ _ _ _ _ _ _ _]
              tunnel: w105 -> [w108 w110 w117 w129 w173 w189 w212 w238 w266 w293 w299 w320 w337 w355 w371 w388 w405 w426 w443 w462 w480 w497 w515 w539 w563 w587 w611 w632 w655 w674 w679 w682 w685 w689 w693 w697 w701 w707 w712 w716 w721 w743 w747 w753 w774 w777 w780 w786 w806]
              tunnel: [w108 w109 w116 w133 w165 w198 w220 w245 w263 w284 w310 w327 w339 w357 w373 w390 w407 w428 w445 w464 w482 w499 w517 w541 w565 w589 w613 w634 w657 w675 w678 w683 w686 w690 w694 w698 w702 w707 w713 w715 w722 w742 w747 w757 w773 w777 w780 w785 w805] -> w104
              tunnel: w103 -> [w107 _ w114 _ _ _ _ _ w262 _ _ _ _ _ _ _ _ _ _ _ _ _ _ _ _ _ _ _ _ w672 w676 w680 w684 w688 w692 w696 w700 w704 w710 w714 w720 w741 w745 w756 w771 w776 w779 w782 w803]
              tunnel: [w107 _ w114 w121 w174 w197 w219 w244 w262 w283 w309 w326 w338 w356 w372 w389 w406 w427 w444 w463 w481 w498 w516 w540 w564 w588 w612 w633 w656 w672 w676 w680 w684 w688 w692 w696 w700 w704 w710 w714 w720 w741 w745 w756 w771 w776 w779 w782 w803] -> w102
              event Timeout {
                n43 = event-data() -> ()  [unwired: 1 in, 3 out]
              }
              event "GPS CMD Send Button": Value Change {
                n44 = event-data() -> ()  [unwired: 1 in, 6 out]
                n45 = local read "GPS serial port"() -> (w111:refnum<visa-resource-name>)
                n46 = call "GPS Input format.vi"("Input"="GPS command input") -> ("Output"=w113:string)
                n47 = VISA Write(VISA resource name=w111, write buffer=w113, error in (no error)=w110) -> (error out=w109:errorcluster)  [unwired: 2 out]
              }
              event "stop": Value Change {
                n48 = event-data() -> ()  [unwired: 1 in, 6 out]
                n49 = call "Append to command queue.vi"("error in (no error)"=w117, "Single command"="Stop") -> ("error out"=w116:errorcluster)  [unwired: 9 in]
              }
              event "Open Master Port", "Open Sniffer Port", "Open ROB Port", "Open GPS Port": Value Change {
                n50 = event-data() -> ("CtlRef"=w119:refnum<vi>)  [unwired: 1 in, 5 out]
                n51 = control-ref of="Open Master Port"() -> (w126:refnum<vi>)
                n52 = control-ref of="Open ROB Port"() -> (w127:refnum<vi>)
                n53 = property class="Bool (strict)"(reference=w119) -> ("Label.Text"=w118:string)  [unwired: 1 in, 2 out]
                n54 = Close Reference(reference=w127, error in (no error)=w129) -> (error out=w128:errorcluster)
                n55 = Close Reference(reference=w126, error in (no error)=w128) -> (error out=w120:errorcluster)
                n56 = case shown="\"Open Master Port\", Default" w118 {
                  tunnel: ["Open Sniffer Port" "Open Master Port" "Open GPS Port" "Open ROB Port"] -> w125
                  tunnel: ["Sniffer serial port" "Master serial port" "GPS serial port" "ROB serial port"] -> w123
                  tunnel: [w146 w149 w152 w159] -> w122
                  tunnel: ["Baud rate sniffer" "Baud rate master" "Baud rate GPS" "Baud rate ROB"] -> w124
                  frame "Open Sniffer Port" {
                    n57 = control-ref of="Sniffer serial port"() -> (w146:refnum<vi>)
                  }
                  frame "Open Master Port", Default {
                    n58 = control-ref of="Master serial port"() -> (w149:refnum<vi>)
                  }
                  frame "Open GPS Port" {
                    n59 = control-ref of="GPS serial port"() -> (w152:refnum<vi>)
                  }
                  frame "Open ROB Port" {
                    n60 = control-ref of="ROB serial port"() -> (w159:refnum<vi>)
                  }
                }
                n61 = case shown="True" w125 {
                  tunnel: w124 -> [_ w141]
                  tunnel: w123 -> [_ w142]
                  tunnel: w122 -> [w134 w143]
                  tunnel: [w135 w137] -> w121
                  frame False {
                    n62 = To Variant(anything=w134) -> (Variant=w136:variant)
                    n63 = Build Array(w136) -> (w135:variant[])
                  }
                  frame True {
                    n64 = To Variant(anything=w143) -> (Variant=w140:variant)
                    n65 = To Variant(anything=w142) -> (Variant=w139:variant)
                    n66 = To Variant(anything=w141) -> (Variant=w138:variant)
                    n67 = Build Array(w140, w139, w138) -> (w137:variant[])
                  }
                }
                n68 = Select(t="OpenSerial", s=w125, f="CloseSerial") -> (s? t:f=w130:string)
                n69 = call "Append to command queue.vi"("error in (no error)"=w120, "Single command"=w130) -> ("error out"=w133:errorcluster)  [unwired: 9 in]
              }
              event "go to standby", "Go to ready", "go to running": Value Change {
                n70 = event-data() -> ("CtlRef"=w169:refnum<vi>)  [unwired: 1 in, 5 out]
                n71 = control-ref of="go to standby"() -> (w171:refnum<vi>)
                n72 = control-ref of="Go to ready"() -> (w170:refnum<vi>)
                n73 = Equal?(x=w170, y=w169) -> (x = y?=w168:bool)
                n74 = Equal?(x=w171, y=w169) -> (x = y?=w172:bool)
                n75 = case shown="False" w172 {
                  tunnel: w168 -> [w179 _]
                  tunnel: [w178 u8 192] -> w167
                  frame False {
                    n76 = case shown="False" w179 {
                      tunnel: [u8 194 u8 193] -> w178
                      frame False {
                      }
                      frame True {
                      }
                    }
                  }
                  frame True {
                  }
                }
                n77 = case shown="16" "Board selector" {
                  selector: "Board selector" -> [_ w185]
                  tunnel: [u8 255 w184] -> w177
                  frame 16 {
                  }
                  frame Default {
                    n78 = To Unsigned Byte Integer(number=w185) -> (unsigned 8bit integer=w184:u8)
                  }
                }
                n79 = call "Append to command queue.vi"("error in (no error)"=w173, "Single command"="SendSerialData") -> ("error out"=w166:errorcluster)  [unwired: 9 in]
                n80 = property on="Master serial port" class="VISAName"(error in=w166) -> (error out=w165:errorcluster, "Value"=w162:refnum<visa-resource-name>)  [unwired: 1 in, 1 out]
                n81 = Build Array(w167, w177) -> (w176:u8[])
                n82 = Byte Array To String(unsigned byte array=w176) -> (string=w175:string)
                n83 = To Variant(anything=w175) -> (Variant=w164:variant)
                n84 = To Variant(anything=w162) -> (Variant=w163:variant)
                n85 = Build Array(w164, w163) -> (w174:variant[])
              }
              event "Set MPPC Bias": Value Change {
                n86 = event-data() -> ()  [unwired: 1 in, 6 out]
                n87 = property on="Board selector" class="Ring (strict)"(error in=w189) -> (error out=w191:errorcluster, "Value"=w196:u16)  [unwired: 1 in, 1 out]
                n88 = case shown="16" w196 {
                  selector: w196 -> [_ w208]
                  tunnel: [u8 255 w207] -> w205
                  frame 16 {
                  }
                  frame Default {
                    n89 = To Unsigned Byte Integer(number=w208) -> (unsigned 8bit integer=w207:u8)
                  }
                }
                n90 = Build Array(u8 176 ("element"), w205, u8 1 ("element")) -> (w204:u8[])
                n91 = Flatten To String(anything="Bias voltage", byte order (0:big-endian, network order)=T19."little-endian", error in (no error)=w191) -> (data string=w192:string, error out=w190:errorcluster)  [unwired: 1 in, 1 out]
                n92 = Byte Array To String(unsigned byte array=w204) -> (string=w193:string)
                n93 = call "Append to command queue.vi"("error in (no error)"=w190, "Single command"="SendSerialData") -> ("error out"=w203:errorcluster)  [unwired: 9 in]
                n94 = property on="Master serial port" class="VISAName"(error in=w203) -> (error out=w198:errorcluster, "Value"=w200:refnum<visa-resource-name>)  [unwired: 1 in, 1 out]
                n95 = Concatenate Strings(w193, w192) -> (w195:string)
                n96 = To Variant(anything=w200) -> (Variant=w201:variant)
                n97 = To Variant(anything=w195) -> (Variant=w202:variant)
                n98 = Build Array(w202, w201) -> (w197:variant[])
              }
              event "Set MPPCovervoltage": Value Change {
                n99 = event-data() -> ()  [unwired: 1 in, 6 out]
                n100 = property on="Board selector" class="Ring (strict)"(error in=w212) -> (error out=w214:errorcluster, "Value"=w218:u16)  [unwired: 1 in, 1 out]
                n101 = case shown="16" w218 {
                  selector: w218 -> [_ w230]
                  tunnel: [u8 255 w229] -> w227
                  frame 16 {
                  }
                  frame Default {
                    n102 = To Unsigned Byte Integer(number=w230) -> (unsigned 8bit integer=w229:u8)
                  }
                }
                n103 = Build Array(u8 178 ("element"), w227) -> (w226:u8[])
                n104 = Flatten To String(anything="Overvoltage", byte order (0:big-endian, network order)=T19."little-endian", error in (no error)=w214) -> (data string=w215:string, error out=w213:errorcluster)  [unwired: 1 in, 1 out]
                n105 = Byte Array To String(unsigned byte array=w226) -> (string=w216:string)
                n106 = call "Append to command queue.vi"("error in (no error)"=w213, "Single command"="SendSerialData") -> ("error out"=w225:errorcluster)  [unwired: 9 in]
                n107 = property on="Master serial port" class="VISAName"(error in=w225) -> (error out=w220:errorcluster, "Value"=w222:refnum<visa-resource-name>)  [unwired: 1 in, 1 out]
                n108 = Concatenate Strings(w216, w215) -> (w217:string)
                n109 = To Variant(anything=w222) -> (Variant=w223:variant)
                n110 = To Variant(anything=w217) -> (Variant=w224:variant)
                n111 = Build Array(w224, w223) -> (w219:variant[])
              }
              event "Set VTrig", "Programmatic set trigthres": Value Change {
                n112 = event-data() -> ()  [unwired: 1 in, 6 out]
                n113 = property on="Board selector" class="Ring (strict)"(error in=w238) -> (error out=w235:errorcluster, "Value"=w243:u16)  [unwired: 1 in, 1 out]
                n114 = case shown="Default" w243 {
                  selector: w243 -> [_ w261]
                  tunnel: [u8 255 w260] -> w252
                  frame 16 {
                  }
                  frame Default {
                    n115 = To Unsigned Byte Integer(number=w261) -> (unsigned 8bit integer=w260:u8)
                  }
                }
                n116 = property on="Hard-set value" class="Bool (strict)"(error in=w235) -> (error out=w234:errorcluster, "Value"=w233:bool)  [unwired: 1 in, 1 out]
                n117 = case shown="True" w233 {
                  tunnel: ["VTrig percent" w256] -> w232
                  tunnel: [u8 2 ("element") u8 1 ("element")] -> w231
                  frame False {
                  }
                  frame True {
                    n118 = Divide(x="VTrig mV", y=sgl 1000.0) -> (x/y=w256:sgl)
                  }
                }
                n119 = Flatten To String(anything=w232, byte order (0:big-endian, network order)=T19."little-endian", error in (no error)=w234) -> (data string=w240:string, error out=w239:errorcluster)  [unwired: 1 in, 1 out]
                n120 = Build Array(u8 177 ("element"), w252, w231) -> (w251:u8[])
                n121 = Byte Array To String(unsigned byte array=w251) -> (string=w241:string)
                n122 = call "Append to command queue.vi"("error in (no error)"=w239, "Single command"="SendSerialData") -> ("error out"=w250:errorcluster)  [unwired: 9 in]
                n123 = property on="Master serial port" class="VISAName"(error in=w250) -> (error out=w245:errorcluster, "Value"=w247:refnum<visa-resource-name>)  [unwired: 1 in, 1 out]
                n124 = Concatenate Strings(w241, w240) -> (w242:string)
                n125 = To Variant(anything=w247) -> (Variant=w248:variant)
                n126 = To Variant(anything=w242) -> (Variant=w249:variant)
                n127 = Build Array(w249, w248) -> (w244:variant[])
              }
              event "Hard-set value": Value Change {
                n128 = event-data() -> ("NewVal"=w267:bool)  [unwired: 1 in, 5 out]
                n129 = case shown="False" w267 {
                  tunnel: [T20."Disabled and Grayed Out" ("Disabled") T20."Enabled" ("Disabled")] -> w268
                  tunnel: [T20."Enabled" ("Disabled") T20."Disabled and Grayed Out" ("Disabled")] -> w265
                  frame False {
                  }
                  frame True {
                  }
                }
                n130 = property on="VTrig mV" class="DigNum (strict)"(error in=w266, "DisabledEnum"=w268) -> (error out=w264:errorcluster)  [unwired: 1 in, 1 out]
                n131 = property on="VTrig percent" class="DigNum (strict)"(error in=w264, "DisabledEnum"=w265) -> (error out=w263:errorcluster)  [unwired: 1 in, 1 out]
              }
              event "Disable auto-VBias": Value Change {
                n132 = event-data() -> ("NewVal"=w273:bool)  [unwired: 1 in, 5 out]
                n133 = case shown="True" w273 {
                  tunnel: [T20."Disabled and Grayed Out" ("Disabled") T20."Enabled" ("Disabled")] -> w291
                  frame False {
                  }
                  frame True {
                  }
                }
                n134 = property on="Set MPPC Bias" class="Bool"(error in=w293, "DisabledEnum"=w291) -> (error out=w292:errorcluster)  [unwired: 1 in, 1 out]
                n135 = property on="Bias voltage" class="DigNum (strict)"(error in=w292, "DisabledEnum"=w291) -> (error out=w276:errorcluster)  [unwired: 1 in, 1 out]
                n136 = property on="Board selector" class="Ring (strict)"(error in=w276) -> (error out=w275:errorcluster, "Value"=w281:u16)  [unwired: 1 in, 1 out]
                n137 = case shown="16" w281 {
                  selector: w281 -> [_ w296]
                  tunnel: [u8 255 w295] -> w280
                  frame 16 {
                  }
                  frame Default {
                    n138 = To Unsigned Byte Integer(number=w296) -> (unsigned 8bit integer=w295:u8)
                  }
                }
                n139 = Select(t=u8 0 ("element"), s=w273, f=u8 1 ("element")) -> (s? t:f=w279:u8)
                n140 = Build Array(u8 245 ("element"), w280, w279) -> (w290:u8[])
                n141 = Byte Array To String(unsigned byte array=w290) -> (string=w274:string)
                n142 = call "Append to command queue.vi"("error in (no error)"=w275, "Single command"="SendSerialData") -> ("error out"=w289:errorcluster)  [unwired: 9 in]
                n143 = property on="Master serial port" class="VISAName"(error in=w289) -> (error out=w284:errorcluster, "Value"=w286:refnum<visa-resource-name>)  [unwired: 1 in, 1 out]
                n144 = To Variant(anything=w286) -> (Variant=w287:variant)
                n145 = To Variant(anything=w274) -> (Variant=w288:variant)
                n146 = Build Array(w288, w287) -> (w283:variant[])
              }
              event "Disable auto latch reset": Value Change {
                n147 = event-data() -> ("NewVal"=w300:bool)  [unwired: 1 in, 5 out]
                n148 = property on="Board selector" class="Ring (strict)"(error in=w299) -> (error out=w302:errorcluster, "Value"=w307:u16)  [unwired: 1 in, 1 out]
                n149 = case shown="16" w307 {
                  selector: w307 -> [_ w319]
                  tunnel: [u8 255 w318] -> w306
                  frame 16 {
                  }
                  frame Default {
                    n150 = To Unsigned Byte Integer(number=w319) -> (unsigned 8bit integer=w318:u8)
                  }
                }
                n151 = Select(t=u8 0 ("element"), s=w300, f=u8 1 ("element")) -> (s? t:f=w305:u8)
                n152 = Build Array(u8 248 ("element"), w306, w305) -> (w316:u8[])
                n153 = Byte Array To String(unsigned byte array=w316) -> (string=w301:string)
                n154 = call "Append to command queue.vi"("error in (no error)"=w302, "Single command"="SendSerialData") -> ("error out"=w315:errorcluster)  [unwired: 9 in]
                n155 = property on="Master serial port" class="VISAName"(error in=w315) -> (error out=w310:errorcluster, "Value"=w312:refnum<visa-resource-name>)  [unwired: 1 in, 1 out]
                n156 = To Variant(anything=w312) -> (Variant=w313:variant)
                n157 = To Variant(anything=w301) -> (Variant=w314:variant)
                n158 = Build Array(w314, w313) -> (w309:variant[])
              }
              event "ROB hard reset": Value Change {
                n159 = event-data() -> ()  [unwired: 1 in, 6 out]
                n160 = property on="Board selector" class="Ring (strict)"(error in=w320) -> (error out=w322:errorcluster, "Value"=w324:u16)  [unwired: 1 in, 1 out]
                n161 = case shown="16" w324 {
                  selector: w324 -> [_ w336]
                  tunnel: [u8 255 w335] -> w323
                  frame 16 {
                  }
                  frame Default {
                    n162 = To Unsigned Byte Integer(number=w336) -> (unsigned 8bit integer=w335:u8)
                  }
                }
                n163 = Build Array(u8 255 ("element"), w323) -> (w333:u8[])
                n164 = Byte Array To String(unsigned byte array=w333) -> (string=w321:string)
                n165 = call "Append to command queue.vi"("error in (no error)"=w322, "Single command"="SendSerialData") -> ("error out"=w332:errorcluster)  [unwired: 9 in]
                n166 = property on="Master serial port" class="VISAName"(error in=w332) -> (error out=w327:errorcluster, "Value"=w329:refnum<visa-resource-name>)  [unwired: 1 in, 1 out]
                n167 = To Variant(anything=w329) -> (Variant=w330:variant)
                n168 = To Variant(anything=w321) -> (Variant=w331:variant)
                n169 = Build Array(w331, w330) -> (w326:variant[])
              }
              event "Rep Temp", "Programmatic rep temp": Value Change {
                n170 = event-data() -> ()  [unwired: 1 in, 6 out]
                n171 = property on="Board selector" class="Ring (strict)"(error in=w337) -> (error out=w341:errorcluster, "Value"=w343:u16)  [unwired: 1 in, 1 out]
                n172 = case shown="16" w343 {
                  selector: w343 -> [_ w353]
                  tunnel: [u8 255 w352] -> w342
                  frame 16 {
                  }
                  frame Default {
                    n173 = To Unsigned Byte Integer(number=w353) -> (unsigned 8bit integer=w352:u8)
                  }
                }
                n174 = Build Array(u8 160 ("element"), w342) -> (w350:u8[])
                n175 = Byte Array To String(unsigned byte array=w350) -> (string=w340:string)
                n176 = call "Append to command queue.vi"("error in (no error)"=w341, "Single command"="SendSerialData") -> ("error out"=w349:errorcluster)  [unwired: 9 in]
                n177 = property on="Master serial port" class="VISAName"(error in=w349) -> (error out=w339:errorcluster, "Value"=w346:refnum<visa-resource-name>)  [unwired: 1 in, 1 out]
                n178 = To Variant(anything=w346) -> (Variant=w347:variant)
                n179 = To Variant(anything=w340) -> (Variant=w348:variant)
                n180 = Build Array(w348, w347) -> (w338:variant[])
              }
              event "Rep voltages", "Programmatic rep volts": Value Change {
                n181 = event-data() -> ()  [unwired: 1 in, 6 out]
                n182 = property on="Board selector" class="Ring (strict)"(error in=w355) -> (error out=w359:errorcluster, "Value"=w361:u16)  [unwired: 1 in, 1 out]
                n183 = case shown="Default" w361 {
                  selector: w361 -> [_ w370]
                  tunnel: [u8 255 w369] -> w360
                  frame 16 {
                  }
                  frame Default {
                    n184 = To Unsigned Byte Integer(number=w370) -> (unsigned 8bit integer=w369:u8)
                  }
                }
                n185 = call "Append to command queue.vi"("error in (no error)"=w359, "Single command"="SendSerialData") -> ("error out"=w366:errorcluster)  [unwired: 9 in]
                n186 = property on="Master serial port" class="VISAName"(error in=w366) -> (error out=w357:errorcluster, "Value"=w354:refnum<visa-resource-name>)  [unwired: 1 in, 1 out]
                n187 = Build Array(u8 161 ("element"), w360) -> (w367:u8[])
                n188 = Byte Array To String(unsigned byte array=w367) -> (string=w358:string)
                n189 = To Variant(anything=w354) -> (Variant=w364:variant)
                n190 = To Variant(anything=w358) -> (Variant=w365:variant)
                n191 = Build Array(w365, w364) -> (w356:variant[])
              }
              event "Rep status", "Programmatic rep stat": Value Change {
                n192 = event-data() -> ()  [unwired: 1 in, 6 out]
                n193 = property on="Board selector" class="Ring (strict)"(error in=w371) -> (error out=w375:errorcluster, "Value"=w377:u16)  [unwired: 1 in, 1 out]
                n194 = case shown="16" w377 {
                  selector: w377 -> [_ w387]
                  tunnel: [u8 255 w386] -> w376
                  frame 16 {
                  }
                  frame Default {
                    n195 = To Unsigned Byte Integer(number=w387) -> (unsigned 8bit integer=w386:u8)
                  }
                }
                n196 = Build Array(u8 162 ("element"), w376) -> (w384:u8[])
                n197 = Byte Array To String(unsigned byte array=w384) -> (string=w374:string)
                n198 = call "Append to command queue.vi"("error in (no error)"=w375, "Single command"="SendSerialData") -> ("error out"=w383:errorcluster)  [unwired: 9 in]
                n199 = property on="Master serial port" class="VISAName"(error in=w383) -> (error out=w373:errorcluster, "Value"=w380:refnum<visa-resource-name>)  [unwired: 1 in, 1 out]
                n200 = To Variant(anything=w380) -> (Variant=w381:variant)
                n201 = To Variant(anything=w374) -> (Variant=w382:variant)
                n202 = Build Array(w382, w381) -> (w372:variant[])
              }
              event "Programmatic rep disclatch", "Rep disclatch": Value Change {
                n203 = event-data() -> ()  [unwired: 1 in, 6 out]
                n204 = property on="Board selector" class="Ring (strict)"(error in=w388) -> (error out=w392:errorcluster, "Value"=w394:u16)  [unwired: 1 in, 1 out]
                n205 = case shown="16" w394 {
                  selector: w394 -> [_ w404]
                  tunnel: [u8 255 w403] -> w393
                  frame 16 {
                  }
                  frame Default {
                    n206 = To Unsigned Byte Integer(number=w404) -> (unsigned 8bit integer=w403:u8)
                  }
                }
                n207 = Build Array(u8 163 ("element"), w393) -> (w401:u8[])
                n208 = Byte Array To String(unsigned byte array=w401) -> (string=w391:string)
                n209 = call "Append to command queue.vi"("error in (no error)"=w392, "Single command"="SendSerialData") -> ("error out"=w400:errorcluster)  [unwired: 9 in]
                n210 = property on="Master serial port" class="VISAName"(error in=w400) -> (error out=w390:errorcluster, "Value"=w397:refnum<visa-resource-name>)  [unwired: 1 in, 1 out]
                n211 = To Variant(anything=w397) -> (Variant=w398:variant)
                n212 = To Variant(anything=w391) -> (Variant=w399:variant)
                n213 = Build Array(w399, w398) -> (w389:variant[])
              }
              event "Rep trigthres": Value Change {
                n214 = event-data() -> ()  [unwired: 1 in, 6 out]
                n215 = property on="Board selector" class="Ring (strict)"(error in=w405) -> (error out=w409:errorcluster, "Value"=w411:u16)  [unwired: 1 in, 1 out]
                n216 = case shown="16" w411 {
                  selector: w411 -> [_ w421]
                  tunnel: [u8 255 w420] -> w410
                  frame 16 {
                  }
                  frame Default {
                    n217 = To Unsigned Byte Integer(number=w421) -> (unsigned 8bit integer=w420:u8)
                  }
                }
                n218 = Build Array(u8 164 ("element"), w410) -> (w418:u8[])
                n219 = Byte Array To String(unsigned byte array=w418) -> (string=w408:string)
                n220 = call "Append to command queue.vi"("error in (no error)"=w409, "Single command"="SendSerialData") -> ("error out"=w417:errorcluster)  [unwired: 9 in]
                n221 = property on="Master serial port" class="VISAName"(error in=w417) -> (error out=w407:errorcluster, "Value"=w414:refnum<visa-resource-name>)  [unwired: 1 in, 1 out]
                n222 = To Variant(anything=w414) -> (Variant=w415:variant)
                n223 = To Variant(anything=w408) -> (Variant=w416:variant)
                n224 = Build Array(w416, w415) -> (w406:variant[])
              }
              event "Remove MPPC": Value Change {
                n225 = event-data() -> ("NewVal"=w425:bool)  [unwired: 1 in, 5 out]
                n226 = property on="Board selector" class="Ring (strict)"(error in=w426) -> (error out=w430:errorcluster, "Value"=w432:u16)  [unwired: 1 in, 1 out]
                n227 = case shown="16" w432 {
                  selector: w432 -> [_ w442]
                  tunnel: [u8 255 w441] -> w431
                  frame 16 {
                  }
                  frame Default {
                    n228 = To Unsigned Byte Integer(number=w442) -> (unsigned 8bit integer=w441:u8)
                  }
                }
                n229 = Select(t=u8 0 ("element"), s=w425, f=u8 1 ("element")) -> (s? t:f=w422:u8)
                n230 = Build Array(u8 208 ("element"), w431, w422) -> (w439:u8[])
                n231 = Byte Array To String(unsigned byte array=w439) -> (string=w429:string)
                n232 = call "Append to command queue.vi"("error in (no error)"=w430, "Single command"="SendSerialData") -> ("error out"=w438:errorcluster)  [unwired: 9 in]
                n233 = property on="Master serial port" class="VISAName"(error in=w438) -> (error out=w428:errorcluster, "Value"=w435:refnum<visa-resource-name>)  [unwired: 1 in, 1 out]
                n234 = To Variant(anything=w435) -> (Variant=w436:variant)
                n235 = To Variant(anything=w429) -> (Variant=w437:variant)
                n236 = Build Array(w437, w436) -> (w427:variant[])
              }
              event "Insert test charge": Value Change {
                n237 = event-data() -> ()  [unwired: 1 in, 6 out]
                n238 = property on="Board selector" class="Ring (strict)"(error in=w443) -> (error out=w447:errorcluster, "Value"=w449:u16)  [unwired: 1 in, 1 out]
                n239 = case shown="16" w449 {
                  selector: w449 -> [_ w459]
                  tunnel: [u8 255 w458] -> w448
                  frame 16 {
                  }
                  frame Default {
                    n240 = To Unsigned Byte Integer(number=w459) -> (unsigned 8bit integer=w458:u8)
                  }
                }
                n241 = Build Array(u8 209 ("element"), w448) -> (w456:u8[])
                n242 = Byte Array To String(unsigned byte array=w456) -> (string=w446:string)
                n243 = call "Append to command queue.vi"("error in (no error)"=w447, "Single command"="SendSerialData") -> ("error out"=w455:errorcluster)  [unwired: 9 in]
                n244 = property on="Master serial port" class="VISAName"(error in=w455) -> (error out=w445:errorcluster, "Value"=w452:refnum<visa-resource-name>)  [unwired: 1 in, 1 out]
                n245 = To Variant(anything=w452) -> (Variant=w453:variant)
                n246 = To Variant(anything=w446) -> (Variant=w454:variant)
                n247 = Build Array(w454, w453) -> (w444:variant[])
              }
              event "Set voltage reference": Value Change {
                n248 = event-data() -> ()  [unwired: 1 in, 6 out]
                n249 = property on="Board selector" class="Ring (strict)"(error in=w462) -> (error out=w466:errorcluster, "Value"=w468:u16)  [unwired: 1 in, 1 out]
                n250 = case shown="16" w468 {
                  selector: w468 -> [_ w478]
                  tunnel: [u8 255 w477] -> w467
                  frame 16 {
                  }
                  frame Default {
                    n251 = To Unsigned Byte Integer(number=w478) -> (unsigned 8bit integer=w477:u8)
                  }
                }
                n252 = To Unsigned Byte Integer(number="Voltage ref") -> (unsigned 8bit integer=w460:u8)
                n253 = Build Array(u8 244 ("element"), w467, w460) -> (w475:u8[])
                n254 = Byte Array To String(unsigned byte array=w475) -> (string=w465:string)
                n255 = call "Append to command queue.vi"("error in (no error)"=w466, "Single command"="SendSerialData") -> ("error out"=w474:errorcluster)  [unwired: 9 in]
                n256 = property on="Master serial port" class="VISAName"(error in=w474) -> (error out=w464:errorcluster, "Value"=w471:refnum<visa-resource-name>)  [unwired: 1 in, 1 out]
                n257 = To Variant(anything=w471) -> (Variant=w472:variant)
                n258 = To Variant(anything=w465) -> (Variant=w473:variant)
                n259 = Build Array(w473, w472) -> (w463:variant[])
              }
              event "Reset latch": Value Change {
                n260 = event-data() -> ("OldVal"=w479:bool)  [unwired: 1 in, 5 out]
                n261 = property on="Reset latch" class="Bool (strict)"("Value"=w479) -> ()  [unwired: 2 in, 2 out]
                n262 = property on="Board selector" class="Ring (strict)"(error in=w480) -> (error out=w484:errorcluster, "Value"=w486:u16)  [unwired: 1 in, 1 out]
                n263 = case shown="16" w486 {
                  selector: w486 -> [_ w496]
                  tunnel: [u8 255 w495] -> w485
                  frame 16 {
                  }
                  frame Default {
                    n264 = To Unsigned Byte Integer(number=w496) -> (unsigned 8bit integer=w495:u8)
                  }
                }
                n265 = Build Array(u8 241 ("element"), w485) -> (w493:u8[])
                n266 = Byte Array To String(unsigned byte array=w493) -> (string=w483:string)
                n267 = call "Append to command queue.vi"("error in (no error)"=w484, "Single command"="SendSerialData") -> ("error out"=w492:errorcluster)  [unwired: 9 in]
                n268 = property on="Master serial port" class="VISAName"(error in=w492) -> (error out=w482:errorcluster, "Value"=w489:refnum<visa-resource-name>)  [unwired: 1 in, 1 out]
                n269 = To Variant(anything=w489) -> (Variant=w490:variant)
                n270 = To Variant(anything=w483) -> (Variant=w491:variant)
                n271 = Build Array(w491, w490) -> (w481:variant[])
              }
              event "Echo": Value Change {
                n272 = event-data() -> ()  [unwired: 1 in, 6 out]
                n273 = property on="Board selector" class="Ring (strict)"(error in=w497) -> (error out=w501:errorcluster, "Value"=w503:u16)  [unwired: 1 in, 1 out]
                n274 = case shown="16" w503 {
                  selector: w503 -> [_ w513]
                  tunnel: [u8 255 w512] -> w502
                  frame 16 {
                  }
                  frame Default {
                    n275 = To Unsigned Byte Integer(number=w513) -> (unsigned 8bit integer=w512:u8)
                  }
                }
                n276 = Build Array(u8 240 ("element"), w502) -> (w510:u8[])
                n277 = Byte Array To String(unsigned byte array=w510) -> (string=w500:string)
                n278 = call "Append to command queue.vi"("error in (no error)"=w501, "Single command"="SendSerialData") -> ("error out"=w509:errorcluster)  [unwired: 9 in]
                n279 = property on="Master serial port" class="VISAName"(error in=w509) -> (error out=w499:errorcluster, "Value"=w506:refnum<visa-resource-name>)  [unwired: 1 in, 1 out]
                n280 = To Variant(anything=w506) -> (Variant=w507:variant)
                n281 = To Variant(anything=w500) -> (Variant=w508:variant)
                n282 = Build Array(w508, w507) -> (w498:variant[])
              }
              event "Set Debug Verbosity": Value Change {
                n283 = event-data() -> ()  [unwired: 1 in, 6 out]
                n284 = property on="Board selector" class="Ring (strict)"(error in=w515) -> (error out=w519:errorcluster, "Value"=w521:u16)  [unwired: 1 in, 1 out]
                n285 = case shown="16" w521 {
                  selector: w521 -> [_ w531]
                  tunnel: [u8 255 w530] -> w520
                  frame 16 {
                  }
                  frame Default {
                    n286 = To Unsigned Byte Integer(number=w531) -> (unsigned 8bit integer=w530:u8)
                  }
                }
                n287 = Build Array(u8 247 ("element"), w520, "Verbosity") -> (w528:u8[])
                n288 = Byte Array To String(unsigned byte array=w528) -> (string=w518:string)
                n289 = call "Append to command queue.vi"("error in (no error)"=w519, "Single command"="SendSerialData") -> ("error out"=w527:errorcluster)  [unwired: 9 in]
                n290 = property on="Master serial port" class="VISAName"(error in=w527) -> (error out=w517:errorcluster, "Value"=w524:refnum<visa-resource-name>)  [unwired: 1 in, 1 out]
                n291 = To Variant(anything=w524) -> (Variant=w525:variant)
                n292 = To Variant(anything=w518) -> (Variant=w526:variant)
                n293 = Build Array(w526, w525) -> (w516:variant[])
              }
              event "Enable 3.3", "Disable 3.3": Value Change {
                n294 = event-data() -> ("CtlRef"=w536:refnum<vi>)  [unwired: 1 in, 5 out]
                n295 = control-ref of="Enable 3.3"() -> (w537:refnum<vi>)
                n296 = Equal?(x=w537, y=w536) -> (x = y?=w535:bool)
                n297 = property on="Board selector" class="Ring (strict)"(error in=w539) -> (error out=w543:errorcluster, "Value"=w545:u16)  [unwired: 1 in, 1 out]
                n298 = case shown="16" w545 {
                  selector: w545 -> [_ w555]
                  tunnel: [u8 255 w554] -> w544
                  frame 16 {
                  }
                  frame Default {
                    n299 = To Unsigned Byte Integer(number=w555) -> (unsigned 8bit integer=w554:u8)
                  }
                }
                n300 = Select(t=u8 1 ("element"), s=w535, f=u8 0 ("element")) -> (s? t:f=w534:u8)
                n301 = To Unsigned Byte Integer(number=w534) -> (unsigned 8bit integer=w538:u8)
                n302 = Build Array(u8 243 ("element"), w544, w538) -> (w552:u8[])
                n303 = Byte Array To String(unsigned byte array=w552) -> (string=w542:string)
                n304 = call "Append to command queue.vi"("error in (no error)"=w543, "Single command"="SendSerialData") -> ("error out"=w551:errorcluster)  [unwired: 9 in]
                n305 = property on="Master serial port" class="VISAName"(error in=w551) -> (error out=w541:errorcluster, "Value"=w548:refnum<visa-resource-name>)  [unwired: 1 in, 1 out]
                n306 = To Variant(anything=w548) -> (Variant=w549:variant)
                n307 = To Variant(anything=w542) -> (Variant=w550:variant)
                n308 = Build Array(w550, w549) -> (w540:variant[])
              }
              event "disable +-5V", "Enable +-5": Value Change {
                n309 = event-data() -> ("CtlRef"=w561:refnum<vi>)  [unwired: 1 in, 5 out]
                n310 = control-ref of="Enable +-5"() -> (w556:refnum<vi>)
                n311 = Equal?(x=w556, y=w561) -> (x = y?=w560:bool)
                n312 = property on="Board selector" class="Ring (strict)"(error in=w563) -> (error out=w567:errorcluster, "Value"=w569:u16)  [unwired: 1 in, 1 out]
                n313 = case shown="16" w569 {
                  selector: w569 -> [_ w579]
                  tunnel: [u8 255 w578] -> w568
                  frame 16 {
                  }
                  frame Default {
                    n314 = To Unsigned Byte Integer(number=w579) -> (unsigned 8bit integer=w578:u8)
                  }
                }
                n315 = Select(t=u8 1 ("element"), s=w560, f=u8 0 ("element")) -> (s? t:f=w559:u8)
                n316 = To Unsigned Byte Integer(number=w559) -> (unsigned 8bit integer=w562:u8)
                n317 = Build Array(u8 242 ("element"), w568, w562) -> (w576:u8[])
                n318 = Byte Array To String(unsigned byte array=w576) -> (string=w566:string)
                n319 = call "Append to command queue.vi"("error in (no error)"=w567, "Single command"="SendSerialData") -> ("error out"=w575:errorcluster)  [unwired: 9 in]
                n320 = property on="Master serial port" class="VISAName"(error in=w575) -> (error out=w565:errorcluster, "Value"=w572:refnum<visa-resource-name>)  [unwired: 1 in, 1 out]
                n321 = To Variant(anything=w572) -> (Variant=w573:variant)
                n322 = To Variant(anything=w566) -> (Variant=w574:variant)
                n323 = Build Array(w574, w573) -> (w564:variant[])
              }
              event "Disable 15", "Enable 15": Value Change {
                n324 = event-data() -> ("CtlRef"=w585:refnum<vi>)  [unwired: 1 in, 5 out]
                n325 = control-ref of="Enable 15"() -> (w580:refnum<vi>)
                n326 = Equal?(x=w580, y=w585) -> (x = y?=w584:bool)
                n327 = property on="Board selector" class="Ring (strict)"(error in=w587) -> (error out=w591:errorcluster, "Value"=w593:u16)  [unwired: 1 in, 1 out]
                n328 = case shown="16" w593 {
                  selector: w593 -> [_ w603]
                  tunnel: [u8 255 w602] -> w592
                  frame 16 {
                  }
                  frame Default {
                    n329 = To Unsigned Byte Integer(number=w603) -> (unsigned 8bit integer=w602:u8)
                  }
                }
                n330 = Select(t=u8 1 ("element"), s=w584, f=u8 0 ("element")) -> (s? t:f=w583:u8)
                n331 = To Unsigned Byte Integer(number=w583) -> (unsigned 8bit integer=w586:u8)
                n332 = Build Array(u8 249 ("element"), w592, w586) -> (w600:u8[])
                n333 = Byte Array To String(unsigned byte array=w600) -> (string=w590:string)
                n334 = call "Append to command queue.vi"("error in (no error)"=w591, "Single command"="SendSerialData") -> ("error out"=w599:errorcluster)  [unwired: 9 in]
                n335 = property on="Master serial port" class="VISAName"(error in=w599) -> (error out=w589:errorcluster, "Value"=w596:refnum<visa-resource-name>)  [unwired: 1 in, 1 out]
                n336 = To Variant(anything=w596) -> (Variant=w597:variant)
                n337 = To Variant(anything=w590) -> (Variant=w598:variant)
                n338 = Build Array(w598, w597) -> (w588:variant[])
              }
              event "Enable amp", "disable amp": Value Change {
                n339 = event-data() -> ("CtlRef"=w609:refnum<vi>)  [unwired: 1 in, 5 out]
                n340 = control-ref of="Enable amp"() -> (w604:refnum<vi>)
                n341 = Equal?(x=w604, y=w609) -> (x = y?=w608:bool)
                n342 = property on="Board selector" class="Ring (strict)"(error in=w611) -> (error out=w615:errorcluster, "Value"=w617:u16)  [unwired: 1 in, 1 out]
                n343 = case shown="16" w617 {
                  selector: w617 -> [_ w627]
                  tunnel: [u8 255 w626] -> w616
                  frame 16 {
                  }
                  frame Default {
                    n344 = To Unsigned Byte Integer(number=w627) -> (unsigned 8bit integer=w626:u8)
                  }
                }
                n345 = Select(t=u8 1 ("element"), s=w608, f=u8 0 ("element")) -> (s? t:f=w607:u8)
                n346 = To Unsigned Byte Integer(number=w607) -> (unsigned 8bit integer=w610:u8)
                n347 = Build Array(u8 246 ("element"), w616, w610) -> (w624:u8[])
                n348 = Byte Array To String(unsigned byte array=w624) -> (string=w614:string)
                n349 = call "Append to command queue.vi"("error in (no error)"=w615, "Single command"="SendSerialData") -> ("error out"=w623:errorcluster)  [unwired: 9 in]
                n350 = property on="Master serial port" class="VISAName"(error in=w623) -> (error out=w613:errorcluster, "Value"=w620:refnum<visa-resource-name>)  [unwired: 1 in, 1 out]
                n351 = To Variant(anything=w620) -> (Variant=w621:variant)
                n352 = To Variant(anything=w614) -> (Variant=w622:variant)
                n353 = Build Array(w622, w621) -> (w612:variant[])
              }
              event "Continuous test charge": Value Change {
                n354 = event-data() -> ()  [unwired: 1 in, 6 out]
                n355 = property on="Board selector" class="Ring (strict)"(error in=w632) -> (error out=w636:errorcluster, "Value"=w638:u16)  [unwired: 1 in, 1 out]
                n356 = case shown="16" w638 {
                  selector: w638 -> [_ w648]
                  tunnel: [u8 255 w647] -> w637
                  frame 16 {
                  }
                  frame Default {
                    n357 = To Unsigned Byte Integer(number=w648) -> (unsigned 8bit integer=w647:u8)
                  }
                }
                n358 = Select(t=u8 1 ("element"), s="Continuous test charge", f=u8 0 ("element")) -> (s? t:f=w631:u8)
                n359 = Build Array(u8 210 ("element"), w637, w631) -> (w645:u8[])
                n360 = Byte Array To String(unsigned byte array=w645) -> (string=w635:string)
                n361 = call "Append to command queue.vi"("error in (no error)"=w636, "Single command"="SendSerialData") -> ("error out"=w644:errorcluster)  [unwired: 9 in]
                n362 = property on="Master serial port" class="VISAName"(error in=w644) -> (error out=w634:errorcluster, "Value"=w641:refnum<visa-resource-name>)  [unwired: 1 in, 1 out]
                n363 = To Variant(anything=w641) -> (Variant=w642:variant)
                n364 = To Variant(anything=w635) -> (Variant=w643:variant)
                n365 = Build Array(w643, w642) -> (w633:variant[])
              }
              event "Disable rail monitor", "enable rail monitor": Value Change {
                n366 = event-data() -> ("CtlRef"=w649:refnum<vi>)  [unwired: 1 in, 5 out]
                n367 = control-ref of="enable rail monitor"() -> (w650:refnum<vi>)
                n368 = property on="Board selector" class="Ring (strict)"(error in=w655) -> (error out=w659:errorcluster, "Value"=w661:u16)  [unwired: 1 in, 1 out]
                n369 = case shown="16" w661 {
                  selector: w661 -> [_ w671]
                  tunnel: [u8 255 w670] -> w660
                  frame 16 {
                  }
                  frame Default {
                    n370 = To Unsigned Byte Integer(number=w671) -> (unsigned 8bit integer=w670:u8)
                  }
                }
                n371 = Equal?(x=w650, y=w649) -> (x = y?=w651:bool)
                n372 = Select(t=u8 1 ("element"), s=w651, f=u8 0 ("element")) -> (s? t:f=w654:u8)
                n373 = Build Array(u8 250 ("element"), w660, w654) -> (w668:u8[])
                n374 = Byte Array To String(unsigned byte array=w668) -> (string=w658:string)
                n375 = call "Append to command queue.vi"("error in (no error)"=w659, "Single command"="SendSerialData") -> ("error out"=w667:errorcluster)  [unwired: 9 in]
                n376 = property on="Master serial port" class="VISAName"(error in=w667) -> (error out=w657:errorcluster, "Value"=w664:refnum<visa-resource-name>)  [unwired: 1 in, 1 out]
                n377 = To Variant(anything=w664) -> (Variant=w665:variant)
                n378 = To Variant(anything=w658) -> (Variant=w666:variant)
                n379 = Build Array(w666, w665) -> (w656:variant[])
              }
              event "Start tdc": Value Change {
                n380 = event-data() -> ()  [unwired: 1 in, 6 out]
                n381 = call "Append to TDC command queue.vi"("error in (no error)"=w674, "Single command"="StartTDC") -> ("error out"=w675:errorcluster)  [unwired: 9 in]
              }
              event "Stop tdc": Value Change {
                n382 = event-data() -> ()  [unwired: 1 in, 6 out]
                n383 = call "Append to TDC command queue.vi"("error in (no error)"=w679, "Single command"="StopTDC") -> ("error out"=w678:errorcluster)  [unwired: 9 in]
              }
              event "Pause tdc": Value Change {
                n384 = event-data() -> ()  [unwired: 1 in, 6 out]
                n385 = call "Append to TDC command queue.vi"("error in (no error)"=w682, "Single command"="PauseTDC") -> ("error out"=w683:errorcluster)  [unwired: 9 in]
              }
              event "Continue tdc": Value Change {
                n386 = event-data() -> ()  [unwired: 1 in, 6 out]
                n387 = call "Append to TDC command queue.vi"("error in (no error)"=w685, "Single command"="ContinueTDC") -> ("error out"=w686:errorcluster)  [unwired: 9 in]
              }
              event "Read Cfg Again": Value Change {
                n388 = event-data() -> ()  [unwired: 1 in, 6 out]
                n389 = call "Append to TDC command queue.vi"("error in (no error)"=w689, "Single command"="ReadCfgFileAgain") -> ("error out"=w690:errorcluster)  [unwired: 9 in]
              }
              event "Get set param names": Value Change {
                n390 = event-data() -> ()  [unwired: 1 in, 6 out]
                n391 = call "Append to TDC command queue.vi"("error in (no error)"=w693, "Single command"="GetParams") -> ("error out"=w694:errorcluster)  [unwired: 9 in]
              }
              event "Reconfigure": Value Change {
                n392 = event-data() -> ()  [unwired: 1 in, 6 out]
                n393 = call "Append to TDC command queue.vi"("error in (no error)"=w697, "Single command"="Reconfigure") -> ("error out"=w698:errorcluster)  [unwired: 9 in]
              }
              event "Read config string": Value Change {
                n394 = event-data() -> ()  [unwired: 1 in, 6 out]
                n395 = call "Append to TDC command queue.vi"("error in (no error)"=w701, "Single command"="ReadCfgString") -> ("error out"=w702:errorcluster)  [unwired: 9 in]
              }
              event "Fast read": Value Change {
                n396 = event-data() -> ("NewVal"=w705:bool)  [unwired: 1 in, 5 out]
                n397 = global read "Global AllowRead.vi" "Global allow TDC read"() -> (w706:bool)
                n398 = case shown="True" w706 {
                  tunnel: w705 -> [_ w708]
                  frame False {
                  }
                  frame True {
                    n399 = Not(x=w708) -> (.not. x?=w709:bool)
                    n400 = global write "AllowTDCHitsRead.vi" "AllowTDCHitsRead"(w709) -> ()
                    n401 = global write "AllowTDCFastRead.vi" "AllowTDCFastRead"(w708) -> ()
                  }
                }
              }
              event "SetMaxHistItems": Value Change {
                n402 = event-data() -> ()  [unwired: 1 in, 6 out]
                n403 = call "Append to command queue.vi"("error in (no error)"=w712, "Single command"="ResizeHistArrays") -> ("error out"=w713:errorcluster)  [unwired: 9 in]
              }
              event "Clear charts": Value Change {
                n404 = event-data() -> ()  [unwired: 1 in, 6 out]
                n405 = call "Append to command queue.vi"("error in (no error)"=w716, "Single command"="ResetCharts") -> ("error out"=w715:errorcluster)  [unwired: 9 in]
              }
              event "Set chart res": Value Change {
                n406 = event-data() -> ()  [unwired: 1 in, 6 out]
                n407 = local read "hit charts refnum cluster"() -> (w719:T12)
                n408 = Cluster To Array(cluster=w719) -> (array=w718:T11[])
                n409 = for {
                  tunnel: w718 -> [w729] mode=indexing
                  shift-right: [w723] -> w722
                  shift-left: w721 -> [w727]
                  stop <- w726 stop-if-true
                  n410 = for {
                    N: 8 -> [_]
                    shift-right: [w733] -> w724
                    shift-left: w727 -> [w739]
                    tunnel: w729 -> [w738]
                    tunnel: [w731] -> w728
                    i -> [w740]
                    n411 = local read "Resolution(seconds)"() -> (w736:dbl)
                    n412 = call "Read chart cluster element.vi"("error in (no error)"=w739, "Chart cluster element"=w740, "Chart cluster"=w738) -> ("error out"=w734:errorcluster, 2:"Chart cluster"=w737:T7, 3:"Chart cluster"=w732:T11)  [unwired: 5 in, 1 out]
                    n413 = Bundle By Name(cluster=w737, "Resolution(s)"=w736) -> (w735:T7)
                    n414 = call "write hitchart data.vi"("Histogram cluster"=w735, "error in (no error)"=w734, "Hit charts"=w732) -> ("error out"=w733:errorcluster, "Hit charts"=w731:T11)  [unwired: 7 in]
                  }
                  n415 = Close Reference(reference=w728) -> (error out=w725:errorcluster)  [unwired: 1 in]
                  n416 = Merge Errors(w725, w724) -> (w723:errorcluster)
                  n417 = Unbundle By Name(w723) -> ("status"=w726:bool)
                }
              }
              event "Master data": Value Change {
                n418 = event-data() -> ()  [unwired: 1 in, 6 out]
                n419 = call "Append to command queue.vi"("error in (no error)"=w743, "Single command"="HandleMasterData") -> ("error out"=w742:errorcluster)  [unwired: 9 in]
              }
              event "Enable usermessages": Value Change {
                n420 = event-data() -> ("NewVal"=w746:bool)  [unwired: 1 in, 5 out]
                n421 = global write "AllowUserMessages.vi" "Allow Usermessages"(w746) -> ()
              }
              event "Start Run": Value Change {
                n422 = event-data() -> ("NewVal"=w754:bool)  [unwired: 1 in, 5 out]
                n423 = control-ref of="GPS serial port"() -> (w752:refnum<vi>)
                n424 = Not(x=w754) -> (.not. x?=w755:bool)
                n425 = global write "AllowUserMessages.vi" "Allow Usermessages"(w755) -> ()
                n426 = property on="Property Node" class="VISAName"(reference=w752, error in=w753) -> (error out=w749:errorcluster, "Value"=w748:refnum<visa-resource-name>)  [unwired: 1 out]
                n427 = Equal?(x=refnum<visa-resource-name> refnum ("Value"), y=w748) -> (x = y?=w750:bool)
                n428 = case shown="True" w754 {
                  tunnel: w749 -> [w760 w763]
                  tunnel: [w759 w762] -> w757
                  tunnel: w750 -> [_ w761]
                  frame False {
                    n429 = call "Append to command queue.vi"("error in (no error)"=w760, "Single command"="StopRun") -> ("error out"=w759:errorcluster)  [unwired: 9 in]
                  }
                  frame True {
                    n430 = case shown="False" w761 {
                      tunnel: w763 -> [w765 w768]
                      tunnel: [w764 w767] -> w762
                      frame False {
                        n431 = call "Append to command queue.vi"("error in (no error)"=w765, "Single command"="StartRun") -> ("error out"=w764:errorcluster)  [unwired: 9 in]
                      }
                      frame True {
                        n432 = One Button Dialog(message="You cannot start a run without first opening the GPS serial port.") -> ()  [unwired: 1 in, 1 out]
                        n433 = property on="Start Run" class="Bool (strict)"(error in=w768, "Value"=FALSE ("Start Run")) -> (error out=w767:errorcluster)  [unwired: 1 in, 1 out]
                      }
                    }
                  }
                }
              }
              event "Open EventDisplay": Value Change {
                n434 = event-data() -> ()  [unwired: 1 in, 6 out]
                n435 = local read "Event display Refnum"() -> (w775:refnum<vi>)
                n436 = invoke class="VI Interface Type 0" method="FP.Open"(reference=w775, error in=w774, "State"=T21."Standard") -> (error out=w773:errorcluster)  [unwired: 2 in, 4 out]
              }
              event "Planar coincidence window": Value Change {
                n437 = event-data() -> ("NewVal"=w778:i32)  [unwired: 1 in, 5 out]
                n438 = global write "Coincidence Windows.vi" "Planar"(w778) -> ()
              }
              event "Coincidence grouping window": Value Change {
                n439 = event-data() -> ("NewVal"=w781:i32)  [unwired: 1 in, 5 out]
                n440 = global write "Coincidence Windows.vi" "CRT-wide"(w781) -> ()
              }
              event "Open trigrate": Value Change {
                n441 = event-data() -> ()  [unwired: 1 in, 6 out]
                n442 = local read "Trig chara refnum"() -> (w783:refnum<vi>)
                n443 = Not A Number/Path/Refnum?(number/path/refnum=w783) -> (NaN/Path/Refnum?=w784:bool)
                n444 = case shown="True" w784 {
                  tunnel: w786 -> [w789 w796]
                  tunnel: [w788 w795] -> w785
                  tunnel: w783 -> [w790 _]
                  frame False {
                    n445 = invoke class="VI Interface Type 1" method="FP.Open"(reference=w790, error in=w789, "Activate"=TRUE ("Activate?")) -> (error out=w788:errorcluster)  [unwired: 2 in, 4 out]
                  }
                  frame True {
                    n446 = vi-ref "Trig Rate Charactarization.vi"() -> (w799:refnum<vi>)
                    n447 = Open VI Reference(type specifier VI Refnum (for type only)=w799, vi path=path "C:/Users/CRT Controller/CRTC Labview Application/Source/VIs/Data taking/Trig Rate Charactarization.vi", options=256, error in (no error)=w796) -> (vi reference=w798:refnum<vi>, error out=w797:errorcluster)  [unwired: 2 in]
                    n448 = control-ref of="Programmatic set trigthres"() -> (w794:refnum<vi>)
                    n449 = control-ref of="VTrig mV"() -> (w792:refnum<vi>)
                    n450 = control-ref of="Reset latch"() -> (w793:refnum<vi>)
                    n451 = call-by-ref "Start Asynchronous Call"(reference=w798, error in=w797, "Reset latch"=w793, 8:"error in (no error)"=w796, "Programmatic set Vtrig"=w794, "VTrig mV"=w792) -> (reference out=→"Trig chara refnum":refnum<vi>, error out=w795:errorcluster)  [unwired: 7 in, 1 out]
                  }
                }
              }
              event "Open coincrate": Value Change {
                n452 = event-data() -> ()  [unwired: 1 in, 6 out]
                n453 = local read "charactirzator refnum"() -> (w802:refnum<vi>)
                n454 = Not A Number/Path/Refnum?(number/path/refnum=w802) -> (NaN/Path/Refnum?=w804:bool)
                n455 = case shown="True" w804 {
                  tunnel: w806 -> [w809 w822]
                  tunnel: [w808 w821] -> w805
                  tunnel: w802 -> [w810 _]
                  frame False {
                    n456 = invoke class="VI (strict)" method="FP.Open"(reference=w810, error in=w809, "Activate"=TRUE ("Activate?")) -> (error out=w808:errorcluster)  [unwired: 2 in, 4 out]
                  }
                  frame True {
                    n457 = control-ref of="VTrig mV"() -> (w819:refnum<vi>)
                    n458 = control-ref of="Programmatic set trigthres"() -> (w820:refnum<vi>)
                    n459 = control-ref of="Top layer hit charts"() -> (w818:refnum<vi>)
                    n460 = control-ref of="Bottom layer hit charts"() -> (w817:refnum<vi>)
                    n461 = control-ref of="Board selector"() -> (w816:refnum<vi>)
                    n462 = control-ref of="VTrig percent"() -> (w814:refnum<vi>)
                    n463 = control-ref of="Hard-set value"() -> (w815:refnum<vi>)
                    n464 = Bundle By Name(cluster=T22 {"VTrig mV"=refnum, "Top hit charts"=refnum, "Bottom hit charts"=refnum, "Board selector"=refnum, "VTrig percent "=refnum, "Hard-set value"=refnum, "Programmatic set trigthres"=refnum} ("Main VI refnums"), "VTrig mV"=w819, "Programmatic set trigthres"=w820, "Top hit charts"=w818, "Bottom hit charts"=w817, "Board selector"=w816, "VTrig percent"=w814, "Hard-set value"=w815) -> (w812:T22)
                    n465 = vi-ref "Characterizator.vi"() -> (w825:refnum<vi>)
                    n466 = Open VI Reference(type specifier VI Refnum (for type only)=w825, vi path=path "C:/Users/CRT Controller/CRTC Labview Application/Source/VIs/Data taking/Coincidence characterizator/Characterizator.vi", options=256, error in (no error)=w822) -> (vi reference=w824:refnum<vi>, error out=w823:errorcluster)  [unwired: 2 in]
                    n467 = call-by-ref "Start Asynchronous Call"(reference=w824, error in=w823, 8:"error in (no error)"=w822, "Main VI refnums"=w812) -> (reference out=→"charactirzator refnum":refnum<vi>, error out=w821:errorcluster)  [unwired: 9 in, 1 out]
                  }
                }
              }
            }
          }
          frame "Initiate" {
            w849 = T20."Disabled and Grayed Out" ("Disabled")
            # "Initialization of the CRTC."
            n468 = property on="Set MPPC Bias" class="Bool"(error in=w853, "DisabledEnum"=w849) -> (error out=w851:errorcluster)  [unwired: 1 in, 1 out]
            n469 = call "1PPS.vi"("Action"=T23."initiate") -> ()  [unwired: 3 in, 1 out]
            n470 = global write "AllowUserMessages.vi" "Allow Usermessages"(TRUE ("Allow Usermessages")) -> ()
            n471 = global write "Coincidence hunt limit.vi" "Coinchunt Lim"(10 ("Coinchunt Lim")) -> ()
            n472 = property on="Bias voltage" class="DigNum (strict)"(error in=w851, "DisabledEnum"=w849) -> (error out=w850:errorcluster)  [unwired: 1 in, 1 out]
            n473 = call "TotalHits.vi"("Number (0)"=u64 0, "Action"=T18."Init") -> ()  [unwired: 9 in, 1 out]
            n474 = call "coincidence stats.vi"("Action"=enum16{"Insert", "Get", "Initiate"}."Initiate") -> ()  [unwired: 8 in, 3 out]
            n475 = property on="VTrig mV" class="DigNum (strict)"(error in=w850, "DisabledEnum"=w849) -> (error out=w848:errorcluster)  [unwired: 1 in, 1 out]
            n476 = global read "System info.vi" "TDCRead Buffer Size"() -> (w834:i32)
            n477 = global read "System info.vi" "Max coinchunt lim"() -> (w833:i32)
            n478 = call "Append to TDC command queue.vi"("error in (no error)"=w848, "Single command"="InitTDC") -> ("error out"=w837:errorcluster)  [unwired: 9 in]
            n479 = call "Append to command queue.vi"("error in (no error)"=w837, "Command Array"=string[] ["LaunchReaders", "LaunchSerials", "LaunchEventDisplay"]) -> ("error out"=w836:errorcluster)  [unwired: 9 in]
            n480 = property on="TDCRead" class="Knob (strict)"("Scale.Maximum"=w834) -> ()  [unwired: 2 in, 2 out]
            n481 = property on="Coincidencehunt limit" class="Knob (strict)"("Scale.Maximum"=w833) -> ()  [unwired: 2 in, 2 out]
            n482 = control-ref of="Histograms cluster"() -> (w847:refnum<vi>)
            n483 = call "Initialize histograms.vi"("Max data elements"="MaxHistItems", "error in"=w836, "Cluster"=w847) -> ("error out"=w843:errorcluster)  [unwired: 8 in]
            n484 = control-ref of="Bottom layer hit charts"() -> (w828:refnum<vi>)
            n485 = control-ref of="Top layer hit charts"() -> (w842:refnum<vi>)
            n486 = call "Initialize hitcharts.vi"("Hit charts bottom"=w828, "Hit charts top"=w842, "error in"=w843, "Resolution(s)"="Resolution(seconds)") -> ("hit charts refnum cluster"=→"hit charts refnum cluster":T12, "error out"=w830:errorcluster)  [unwired: 10 in]
            n487 = flat-sequence {
              tunnel: w830 -> [w855]
              tunnel: [w855] -> w829
              frame #0 {
                "Initiate finished" <- TRUE
              }
            }
          }
          frame "LaunchSerials" {
            # "Launches asynchronous Serial readers and the Master command sender"
            n488 = control-ref of="Master Serial Input Data"() -> (w884:refnum<vi>)
            n489 = control-ref of="Master serial port"() -> (w886:refnum<vi>)
            n490 = control-ref of="Master data"() -> (w885:refnum<vi>)
            n491 = control-ref of="ROB serial port"() -> (w881:refnum<vi>)
            n492 = control-ref of="ROB Serial Input Data"() -> (w880:refnum<vi>)
            n493 = control-ref of="Sniffer serial port"() -> (w877:refnum<vi>)
            n494 = control-ref of="Sniffer Serial Input Data"() -> (w876:refnum<vi>)
            n495 = control-ref of="GPS serial port"() -> (w861:refnum<vi>)
            n496 = control-ref of="GPS serial input data"() -> (w860:refnum<vi>)
            n497 = Bundle By Name(cluster=T24 {"VISAResourceName in"=refnum, "Input buffer refnum"=refnum} ("ROB Serial cluster"), "VISAResourceName in"=w881, "Input buffer refnum"=w880) -> (w879:T24)
            n498 = Bundle By Name(cluster=T25 {"Master data ref"=refnum, "VISAResourceName in"=refnum, "Input buffer refnum"=refnum} ("Master serial cluster"), "Master data ref"=w885, "VISAResourceName in"=w886, "Input buffer refnum"=w884) -> (w883:T25)
            n499 = Bundle By Name(cluster=T24 {"VISAResourceName in"=refnum, "Input buffer refnum"=refnum} ("Sniffer serial cluster"), "VISAResourceName in"=w861, "Input buffer refnum"=w860) -> (w858:T24)
            n500 = Bundle By Name(cluster=T24 {"VISAResourceName in"=refnum, "Input buffer refnum"=refnum} ("Sniffer serial cluster"), "VISAResourceName in"=w877, "Input buffer refnum"=w876) -> (w875:T24)
            n501 = call "Asyncronous launcher.vi"("Master serial cluster"=w883, "ROB Serial cluster"=w879, "GPS Serial cluster"=w858, "Sniffer serial cluster"=w875, "error in"=w874) -> ("MasterSerial Refnum"=→"MasterSerial Refnum":refnum<vi>, "SnifferSerial Refnum"=→"SnifferSerial Refnum":refnum<vi>, "GPSSerial Refnum"=→"GPSSerial Refnum":refnum<vi>, "ROBSerial Refnum"=→"ROBSerial Refnum":refnum<vi>, "error out"=w865:errorcluster)  [unwired: 6 in]
            n502 = vi-ref "SendCommands.vi"() -> (w868:refnum<vi>)
            n503 = Open VI Reference(type specifier VI Refnum (for type only)=w868, vi path=path "C:/Users/CRT Controller/CRTC Labview Application/Source/VIs/Serial/SendCommands.vi", options=256, error in (no error)=w865) -> (vi reference=w867:refnum<vi>, error out=w866:errorcluster)  [unwired: 2 in]
            n504 = call-by-ref "Start Asynchronous Call"(reference=w867, error in=w866, 8:"error in (no error)"=w865) -> (reference out=→"Master command sender refnum":refnum<vi>, error out=w864:errorcluster)  [unwired: 10 in, 1 out]
          }
          frame "LaunchReaders" {
            # "Launches asynchronous TDCHit readers and the TDCHit sorter."
            n505 = control-ref of="Sorter overflow"() -> (w897:refnum<vi>)
            n506 = control-ref of="TDCRead overflow"() -> (w895:refnum<vi>)
            n507 = control-ref of="Coinchunt overflow"() -> (w892:refnum<vi>)
            n508 = control-ref of="TDCManager"() -> (w888:refnum<vi>)
            n509 = Bundle By Name(cluster=T27 {"TDCManager Refnum"=refnum, "Unable to keep up indicator"=refnum} ("FastRead cluster"), "TDCManager Refnum"=w888, "Unable to keep up indicator"=w895) -> (w893:T27)
            n510 = Bundle By Name(cluster=T28 {"TDCManager Refnum"=refnum, "Queue overflow indicator"=refnum, "Hit rate warning"=refnum} ("Read Cluster"), "TDCManager Refnum"=w888, "Queue overflow indicator"=w897, "Hit rate warning"=w895) -> (w894:T28)
            n511 = call "Asyncronous TDCReader launcher.vi"("error in"=w901, "hitRateWarning ChannelHits"=w892, "FastRead cluster"=w893, "Read Cluster"=w894) -> ("error out"=w900:errorcluster, "Sorter Refnum"=→"Sorter Refnum":refnum<vi>, "TDCFastRead Refnum"=→"TDCFastRead Refnum":refnum<vi>, "TDCRead Refnum"=→"TDCRead Refnum":refnum<vi>)  [unwired: 4 in]
          }
          frame "LaunchEventDisplay" {
            n512 = vi-ref "EventDisplayWindow.vi"() -> (w908:refnum<vi>)
            n513 = Open VI Reference(type specifier VI Refnum (for type only)=w908, vi path=path "C:/Users/CRT Controller/CRTC Labview Application/Source/VIs/Event display/EventDisplayWindow.vi", options=256, error in (no error)=w910) -> (vi reference=w905:refnum<vi>, error out=w912:errorcluster)  [unwired: 2 in]
            n514 = property class="VI Interface Type 0"(reference=w905, "Exec.ShowFPOnCall"=FALSE ("Execution:Show Front Panel On Call")) -> (reference out=w904:refnum<vi>)  [unwired: 1 in, 1 out]
            n515 = call-by-ref "Start Asynchronous Call"(reference=w904, error in=w912, 8:"error in (no error)"=w910, "Path to detector WRL file"=path "C:/Users/CRT Controller/CRTC Labview Application/Source/Configurations etc/Eventdisplay Geometry.wrl") -> (reference out=→"Event display Refnum":refnum<vi>, error out=w911:errorcluster)  [unwired: 9 in, 1 out]
          }
          frame "TimeOut" {
            n516 = call "Display Message to User"("Message"="Queue Timeout!" ("string")) -> ()  [unwired: 9 in, 2 out]
          }
          frame "Stop" {
            w931 = "Stop" ("Single command")
            w951 = "CommandQueue" ("name (unnamed)")
            # "We flush the command queue and stop the state machine"
            n517 = property on="StopNotifier" class="TypRef (strict)"() -> (error out=w948:errorcluster, "Value"=w949:refnum<notifier>)  [unwired: 2 in, 1 out]
            n518 = property on="GPS serial port" class="VISAName"() -> (error out=w919:errorcluster, "Value"=w920:refnum<visa-resource-name>)  [unwired: 2 in, 1 out]
            n519 = property on="Master serial port" class="VISAName"() -> (error out=w944:errorcluster, "Value"=w945:refnum<visa-resource-name>)  [unwired: 2 in, 1 out]
            n520 = property on="Sniffer serial port" class="VISAName"() -> (error out=w946:errorcluster, "Value"=w941:refnum<visa-resource-name>)  [unwired: 2 in, 1 out]
            n521 = property on="ROB serial port" class="VISAName"() -> (error out=w942:errorcluster, "Value"=w943:refnum<visa-resource-name>)  [unwired: 2 in, 1 out]
            n522 = Obtain Queue(name (unnamed)=w951, element data type=w951, error in (no error)=w950) -> (queue out=w954:refnum<queue>, error out=w953:errorcluster)  [unwired: 2 in, 1 out]
            n523 = call "Close serial.vi"("error in (no error)"=w944, "VISA name"=w945) -> ("error out"=w939:errorcluster)  [unwired: 9 in]
            n524 = call "Close serial.vi"("error in (no error)"=w942, "VISA name"=w943) -> ("error out"=w937:errorcluster)  [unwired: 9 in]
            n525 = Send Notification(notification=TRUE, notifier=w949, error in (no error)=w948) -> (error out=w940:errorcluster)  [unwired: 1 out]
            n526 = call "Close serial.vi"("error in (no error)"=w946, "VISA name"=w941) -> ("error out"=w938:errorcluster)  [unwired: 9 in]
            n527 = call "Close serial.vi"("error in (no error)"=w919, "VISA name"=w920) -> ("error out"=w917:errorcluster)  [unwired: 9 in]
            n528 = Release Queue(queue=w954, force destroy? (F)=TRUE, error in (no error)=w953) -> (error out=w918:errorcluster)  [unwired: 2 out]
            n529 = call "Append to TDC command queue.vi"("Single command"=w931) -> ("error out"=w936:errorcluster)  [unwired: 10 in]
            n530 = call "Append to command queue.vi"("Name (CommandQueue)"="TCQ" ("Single command"), "Single command"=w931) -> ("error out"=w935:errorcluster)  [unwired: 9 in]
            n531 = call "Append to command queue.vi"("Name (CommandQueue)"="CoincChara" ("Single command"), "Single command"=w931) -> ("error out"=w932:errorcluster)  [unwired: 9 in]
            n532 = Merge Errors(w932, w935, w936, w940, w939, w938, w937, w917, w918) -> (w924:errorcluster)
            n533 = call <vilib>:"Stop Timed Structure.vi"("name"="hitratechecker") -> ("error out"=w921:errorcluster)  [unwired: 10 in]
            n534 = call <vilib>:"Stop Timed Structure.vi"("name"="autoreadtimer") -> ("error out"=w925:errorcluster)  [unwired: 10 in]
            n535 = call <vilib>:"Stop Timed Structure.vi"("name"="DayChecker") -> ("error out"=w926:errorcluster)  [unwired: 10 in]
            n536 = Merge Errors(w921, w925, w926, w924) -> (w923:errorcluster)
            n537 = global write "AllowTDCHitsRead.vi" "AllowTDCHitsRead"(FALSE ("AllowTDCHitsRead")) -> ()
            n538 = global write "Global AllowRead.vi" "Global allow TDC read"(FALSE ("AllowRead")) -> ()
          }
          frame Default {
            n539 = Concatenate Strings(w959, " is not valid command for state machine." ("string")) -> (w960:string)
            n540 = call "Display Message to User2"("Message"=w960) -> ()  [unwired: 9 in, 2 out]
          }
          frame "OpenSerial" {
            # "Opens a serial port. Takes three variables: \n1: Refnum to VISA indicator that will hold the opened port\n2: VISA name of the port you wish to open.\n3: Baud rate."
            n541 = Index Array(array=w988, index #1=0 ("index"), index #2=1 ("index"), index #3=2 ("index")) -> (element #1=w984:variant, element #2=w982:variant, element #3=w980:variant)
            n542 = Variant To Data(error in=w976, type=refnum<vi> refnum ("Serial port 1"), Variant=w984) -> (data=w967:refnum<vi>, error out=w978:errorcluster)
            n543 = Variant To Data(error in=w978, type=refnum<visa-resource-name> refnum ("Master serial port"), Variant=w982) -> (data=w971:refnum<visa-resource-name>, error out=w977:errorcluster)
            n544 = Variant To Data(error in=w977, type=u32 0 ("baud rate"), Variant=w980) -> (data=w970:u32, error out=w975:errorcluster)
            n545 = call-poly "VISA Configure Serial Port"("VISA resource name"=w971, "timeout (10sec)"=u32 1000, "baud rate (9600)"=w970, "error in (no error)"=w975) -> ("VISA resource name out"=w965:refnum<visa-resource-name>, "error out"=w963:errorcluster)  [unwired: 10 in]
            n546 = flat-sequence {
              tunnel: w967 -> [w993]
              tunnel: [w993] -> w966
              tunnel: [w992] -> w964
              tunnel: w965 -> [w992]
              tunnel: [w991] -> w962
              tunnel: w963 -> [w991]
              frame #0 {
                n547 = Wait (ms)(milliseconds to wait=u32 100) -> ()  [unwired: 1 out]
              }
            }
            n548 = VISA Flush I/O Buffer(VISA resource name=w964, error in (no error)=w962) -> (VISA resource name out=w969:refnum<visa-resource-name>, error out=w968:errorcluster)  [unwired: 1 in]
            n549 = property class="VISAName"(reference=w966, error in=w968, "Value"=w969) -> (reference out=w973:refnum<vi>, error out=w972:errorcluster)
            n550 = Close Reference(reference=w973, error in (no error)=w972) -> (error out=w974:errorcluster)
          }
          frame "CloseSerial" {
            # "Closes serial port. Takes 1 variable:\n1: Refnum to VISA indicator that contains the port to close."
            n551 = Index Array(array=w1009, index=0) -> (element=w1007:variant)
            n552 = Variant To Data(error in=w1006, type=refnum<vi> refnum ("Serial port 1"), Variant=w1007) -> (data=w1005:refnum<vi>, error out=w1004:errorcluster)
            n553 = property class="VISAName"(reference=w1005, error in=w1004) -> (reference out=w1003:refnum<vi>, error out=w995:errorcluster, "Value"=w996:refnum<visa-resource-name>)
            n554 = VISA Flush I/O Buffer(VISA resource name=w996, error in (no error)=w995) -> (VISA resource name out=w997:refnum<visa-resource-name>, error out=w994:errorcluster)  [unwired: 1 in]
            n555 = VISA Close(VISA resource name=w997, error in (no error)=w994) -> (error out=w1002:errorcluster)
            n556 = invoke class="VISAName" method="Reinit To Default"(reference=w1003, error in=w1002) -> (reference out=w1001:refnum<vi>, error out=w1000:errorcluster)  [unwired: 1 in, 1 out]
            n557 = Close Reference(reference=w1001, error in (no error)=w1000) -> (error out=w999:errorcluster)
          }
          frame "SendSerialData" {
            # "If data is sent to the master we need to listen  for an acknowledgement"
            # "Sends data over a serial port. Takes two arguments:\n1: String consisting of data to send.\n2: Serial port VISA name to send the data over."
            n558 = Index Array(array=w1027, index #1=0 ("index"), index #2=1 ("index")) -> (element #1=w1019:variant, element #2=w1022:variant)
            n559 = local read "Master serial port"() -> (w1018:refnum<visa-resource-name>)
            n560 = Variant To Data(error in=w1020, type=refnum<visa-resource-name> refnum ("Master serial port"), Variant=w1022) -> (data=w1012:refnum<visa-resource-name>, error out=w1023:errorcluster)
            n561 = Equal?(x=w1018, y=w1012) -> (x = y?=w1017:bool)
            n562 = disable-structure shown="Enabled" {
              disable-tunnel: w1019 -> [w1029 _]
              disable-tunnel: w1017 -> [w1028 _]
              frame Disabled {
                n563 = case shown="True" w1028 {
                  tunnel: w1029 -> [_ w1030]
                  frame False {
                  }
                  frame True {
                    n564 = Tick Count (ms)() -> (millisecond timer value=w1033:u32)
                    n565 = while {
                      tunnel: [w1054] -> w1031
                      tunnel: w1033 -> [w1052]
                      tunnel: [w1047] -> w1032
                      stop <- w1049 stop-if-true
                      n566 = event shown="[1] \"Master data\": Value Change" {
                        selector: _ -> [_ _]
                        dyn-events: _ -> [_ _]
                        timeout: 20 -> [_ _]
                        tunnel: [_ w1057] -> w1048
                        tunnel: [_ w1056] -> w1054
                        event Timeout {
                          n567 = event-data() -> ()  [unwired: 1 in, 3 out]
                        }
                        event "Master data": Value Change {
                          n568 = event-data() -> ("NewVal"=w1058:u8[][])  [unwired: 1 in, 4 out]
                          n569 = for {
                            tunnel: w1058 -> [w1063] mode=indexing
                            tunnel: [w1061] -> w1057
                            tunnel: [w1060] -> w1056
                            stop <- w1061 stop-if-true
                            n570 = call "Combine.vi"("NewVal"=w1063) -> ("Data"=w1064:u8[])  [unwired: 10 in]
                            n571 = call "For ROB cluster.vi"("Data in"=w1064) -> ("Type"=w1062:enum16{"ROB info", "Error/Success", "Transm."}, "Data out"=w1059:u8[])  [unwired: 9 in]
                            n572 = case shown="Default" w1062 {
                              tunnel: w1059 -> [_ w1072]
                              tunnel: [_ w1066] -> w1061
                              tunnel: [_ w1065] -> w1060
                              frame Default {
                              }
                              frame "Transm." {
                                n573 = Index Array(array=w1072, index=3) -> (element=w1065:u8)
                                n574 = Equal?(x=w1065, y=u8 1) -> (x = y?=w1067:bool)
                                n575 = Equal?(x=w1065, y=u8 0) -> (x = y?=w1068:bool)
                                n576 = Or(x=w1068, y=w1067) -> (x .or. y?=w1066:bool)
                              }
                            }
                          }
                        }
                      }
                      n577 = Tick Count (ms)() -> (millisecond timer value=w1053:u32)
                      n578 = Subtract(x=w1053, y=w1052) -> (x-y=w1051:u32)
                      n579 = Greater?(x=w1051, y=u32 500) -> (0:w1047:bool)
                      n580 = Or(x=w1048, y=w1047) -> (x .or. y?=w1049:bool)
                    }
                    n581 = case shown="True" w1032 {
                      tunnel: w1031 -> [w1035 _]
                      tunnel: w1030 -> [w1034 _]
                      frame False {
                        n582 = case shown="1" w1035 {
                          tunnel: w1034 -> [_ w1036]
                          frame 0, Default {
                            # "Master recognized packet"
                          }
                          frame 1 {
                            n583 = Variant To Data(type=u8[] [], Variant=w1036) -> (data=w1039:u8[])  [unwired: 1 in, 1 out]
                            n584 = Number To Hexadecimal String(1:i16 2 ("width (-)"), 2:w1039) -> (0:w1042:string[])
                            n585 = for {
                              shift-right: [w1045] -> w1037
                              shift-left: "A command was sent to the master, but the master did not acknowledge it. The data sent was:\n" -> [w1046]
                              tunnel: w1042 -> [w1044] mode=indexing
                              n586 = Concatenate Strings(w1046, w1044, " " ("string")) -> (w1045:string)
                            }
                            n587 = call "Display Message to User8"("Message"=w1037) -> ()  [unwired: 9 in, 2 out]
                          }
                        }
                      }
                      frame True {
                        n588 = call "Display Message to User7"() -> ()  [unwired: 10 in, 2 out]
                      }
                    }
                  }
                }
              }
              frame Enabled {
              }
            }
            n589 = Variant To Data(error in=w1023, type="", Variant=w1019) -> (data=w1013:string, error out=w1016:errorcluster)
            n590 = local read "MasterCmdQueue"() -> (w1015:refnum<queue>)
            n591 = Bundle(cluster=T13 {"Data"="", "Port"=""} ("element"), "Data"=w1013, "Port"=w1012) -> (w1011:T13)
            n592 = Enqueue Element(queue=w1015, element=w1011, error in (no error)=w1016) -> (error out=w1010:errorcluster)  [unwired: 1 in, 2 out]
          }
          frame "ResizeHistArrays" {
            n593 = call <vilib>:"Obtain Semaphore Reference.vi"("error in (no error)"=w1081, "name (unnamed)"="HistSem") -> ("error out"=w1083:errorcluster, "semaphore"=w1084:T29)  [unwired: 3 in, 1 out]
            n594 = call <vilib>:"Acquire Semaphore.vi"("error in (no error)"=w1083, "ms timeout (-1)"=100, "semaphore"=w1084) -> ("error out"=w1079:errorcluster, "timed out"=w1080:bool, "semaphore out"=w1078:T29)  [unwired: 2 in]
            n595 = case shown="False" w1080 {
              tunnel: w1079 -> [w1090 w1105]
              tunnel: w1078 -> [w1088 w1106]
              tunnel: [w1087 w1105] -> w1075
              tunnel: [w1086 w1106] -> w1077
              frame False {
                n596 = property on="MaxHistItems" class="DigNum (strict)"(error in=w1090) -> (error out=w1091:errorcluster, "Value"=w1093:i32)  [unwired: 1 in, 1 out]
                n597 = control-ref of="Histograms cluster"() -> (w1094:refnum<vi>)
                n598 = flat-sequence {
                  tunnel: w1094 -> [w1099]
                  tunnel: w1093 -> [w1098]
                  tunnel: "Histogram select" -> [w1097]
                  tunnel: w1091 -> [w1096]
                  tunnel: [w1095] -> w1089
                  tunnel: w1089 -> [w1103]
                  tunnel: w1088 -> [w1104]
                  tunnel: [w1101] -> w1087
                  tunnel: [w1100] -> w1086
                  frame #0 {
                    n599 = call "Resize hist cluster rolling array.vi"("error in (no error)"=w1096, "Enum"=w1097, "Max number of elements"=w1098, "Cluster"=w1099) -> ("error out"=w1095:errorcluster)  [unwired: 7 in]
                  }
                  frame #1 {
                    n600 = call <vilib>:"Release Semaphore.vi"("semaphore"=w1104) -> ("error out"=w1102:errorcluster, "semaphore out"=w1100:T29)  [unwired: 5 in]
                    n601 = Merge Errors(w1102, w1103) -> (w1101:errorcluster)
                  }
                }
              }
              frame True {
              }
            }
            n602 = call <vilib>:"Release Semaphore Reference.vi"("semaphore"=w1077) -> ("error out"=w1076:errorcluster)  [unwired: 9 in, 1 out]
            n603 = Merge Errors(w1076, w1075) -> (w1074:errorcluster)
          }
          frame "StartRun" {
            n604 = call "Update run counter file.vi"("error in (no error)"=w1112, "run counter path"="run counter path") -> ("error out"=w1110:errorcluster, "Run ID"=w1109:i32, "Process cancelled"=w1111:bool)  [unwired: 7 in]
            n605 = case shown="False" w1111 {
              tunnel: w1110 -> [w1122 w1131]
              tunnel: w1109 -> [w1120 _]
              tunnel: [w1119 w1131] -> w1108
              frame False {
                n606 = call "Open Weekly Save File.vi"("error in (no error)"=w1122, "Data recording root path"="Data recording root path") -> ("error out"=w1121:errorcluster, "Daily datafile"=w1123:T10)  [unwired: 8 in]
                n607 = Get Date/Time In Seconds() -> (seconds since 1Jan1904=→"Run initiated at":timestamp)
                n608 = call "Build new run group.vi"("error in (no error)"=w1121, "Run ID"=w1120, "Daily datafile"=w1123) -> ("error out"=w1115:errorcluster, "Daily datafile"=w1114:T10)  [unwired: 7 in]
                n609 = flat-sequence {
                  tunnel: w1115 -> [w1126]
                  tunnel: [w1126] -> w1118
                  tunnel: w1114 -> [w1125]
                  tunnel: w1118 -> [w1128]
                  tunnel: [w1128] -> w1117
                  tunnel: [w1129] -> w1119
                  tunnel: w1117 -> [w1129]
                  frame #0 {
                    "Daily datafile reference" <- w1125
                  }
                  frame #1 {
                    n610 = Wait (ms)(milliseconds to wait=u32 100) -> ()  [unwired: 1 out]
                  }
                  frame #2 {
                    n611 = global write "take CRT data.vi" "Save CRT data"(TRUE ("Save CRT data")) -> ()
                  }
                }
                "Run ID" <- w1120
              }
              frame True {
                n612 = call "Display Message to User9"("Message"="An eccor occured when trying to update the run counter. Please ensure that the run counter path (in the \"low level\" tab) is correct, and that you have read and write access to this folder.") -> ()  [unwired: 9 in, 2 out]
              }
            }
          }
          frame "SwitchFiles" {
            n613 = stacked-sequence {
              seq-local: [w1137 _ _ _ _ _ _ _] -> [_ w1139 _ _ _ _ _ _]
              seq-local: [_ w1139 _ _ _ _ _ _] -> [_ _ w1141 _ _ _ _ _]
              seq-local: [_ _ w1141 _ _ _ _ _] -> [_ _ _ _ _ w1149 _ _]
              seq-local: [_ _ _ _ _ w1148 _ _] -> [_ _ _ _ _ _ w1153 _]
              seq-local: [_ _ _ _ _ _ w1153 _] -> [_ _ _ _ _ _ _ w1155]
              tunnel: w1135 -> [w1137 _ _ _ _ _ _ _]
              tunnel: [_ _ _ _ _ _ _ w1155] -> w1134
              frame #0 {
                n614 = global write "take CRT data.vi" "File switch"(TRUE ("Save CRT data")) -> ()
              }
              frame #1 {
                n615 = Wait (ms)(milliseconds to wait=u32 250) -> ()  [unwired: 1 out]
              }
              frame #2 {
                n616 = global write "take CRT data.vi" "Save CRT data"(FALSE ("Save CRT data")) -> ()
              }
              frame #3 {
                n617 = Wait (ms)(milliseconds to wait=u32 250) -> ()  [unwired: 1 out]
              }
              frame #4 {
                n618 = local read "Daily datafile reference"() -> (w1143:T10)
                n619 = call <vilib>:"H5Fclose.vi"("ref"=w1143) -> ()  [unwired: 10 in, 1 out]
              }
              frame #5 {
                n620 = local read "Data recording root path"() -> (w1147:path)
                n621 = local read "Planar coincidence window"() -> (w1144:i32)
                n622 = local read "Run ID"() -> (w1146:i32)
                n623 = call "Open Weekly Save File.vi"("error in (no error)"=w1149, "Data recording root path"=w1147) -> ("error out"=w1150:errorcluster, "Daily datafile"=w1151:T10)  [unwired: 8 in]
                n624 = call "Build new run group.vi"("error in (no error)"=w1150, "Numeric"=w1144, "Run ID"=w1146, "Daily datafile"=w1151) -> ("error out"=w1148:errorcluster, "Daily datafile"=w1145:T10)  [unwired: 6 in]
                n625 = local write "Daily datafile reference"(w1145) -> ()
              }
              frame #6 {
                n626 = Wait (ms)(milliseconds to wait=u32 250) -> ()  [unwired: 1 out]
              }
              frame #7 {
                n627 = global write "take CRT data.vi" "Save CRT data"(TRUE ("Save CRT data")) -> ()
              }
            }
          }
          frame "StopRun" {
            n628 = global read "take CRT data.vi" "Save CRT data"() -> (w1159:bool)
            n629 = case shown="False" w1159 {
              tunnel: w1158 -> [w1160 w1164]
              tunnel: [w1160 w1163] -> w1157
              frame False {
              }
              frame True {
                n630 = flat-sequence {
                  tunnel: w1164 -> [w1166]
                  tunnel: [w1166] -> w1162
                  tunnel: w1162 -> [w1168]
                  tunnel: [w1168] -> w1161
                  tunnel: [w1169] -> w1163
                  tunnel: w1161 -> [w1170]
                  frame #0 {
                    n631 = global write "take CRT data.vi" "Save CRT data"(FALSE ("Save CRT data")) -> ()
                  }
                  frame #1 {
                    n632 = Wait (ms)(milliseconds to wait=u32 100) -> ()  [unwired: 1 out]
                  }
                  frame #2 {
                    n633 = local read "Daily datafile reference"() -> (w1171:T10)
                    n634 = call <vilib>:"H5Fclose.vi"("error in (no error)"=w1170, "ref"=w1171) -> ("error out"=w1169:errorcluster)  [unwired: 9 in]
                  }
                }
              }
            }
          }
          frame "HandleMasterData" {
            n635 = control-ref of="Master data"() -> (w1176:refnum<vi>)
            n636 = call "ReadMasterData.vi"("error in (no error)"=w1177, "Array in"=w1176) -> ("error out"=w1174:errorcluster, "Data"=w1175:u8[][])  [unwired: 8 in]
            n637 = for {
              tunnel: w1175 -> [w1180] mode=indexing
              shift-right: [w1178] -> w1173
              shift-left: w1174 -> [w1179]
              n638 = Array Size(array=w1180) -> (size(s)=w1184:i32)
              n639 = Quotient & Remainder(x=w1184, y=2) -> (x-y*floor(x/y)=w1182:i32)  [unwired: 1 out]
              n640 = Equal To 0?(x=w1182) -> (x = 0?=w1181:bool)
              n641 = case shown="True" w1181 {
                tunnel: w1180 -> [_ w1194]
                tunnel: w1179 -> [w1188 w1192]
                tunnel: [w1187 w1191] -> w1178
                frame False {
                  n642 = global read "AllowUserMessages.vi" "Allow Usermessages"() -> (w1186:bool)
                  n643 = call "Display Message to User6"("error in (no error)"=w1188, "Enable"=w1186) -> ("error out"=w1187:errorcluster, "OK"=w1185:bool)  [unwired: 8 in]
                  n644 = global write "AllowUserMessages.vi" "Allow Usermessages"(w1185) -> ()
                }
                frame True {
                  n645 = call "Combine.vi"("NewVal"=w1194) -> ("Data"=w1193:u8[])  [unwired: 10 in]
                  n646 = control-ref of="ROB Info cluster"() -> (w1190:refnum<vi>)
                  n647 = call "For ROB cluster.vi"("Data in"=w1193) -> ("Type"=w1189:enum16{"ROB info", "Error/Success", "Transm."}, "Data out"=w1195:u8[])  [unwired: 9 in]
                  n648 = case shown="\"ROB info\", Default" w1189 {
                    tunnel: w1195 -> [w1199 w1203 w1206]
                    tunnel: w1192 -> [w1198 w1202 w1204]
                    tunnel: [w1197 w1201 w1205] -> w1191
                    tunnel: w1190 -> [w1196 w1200 w1207]
                    frame "ROB info", Default {
                      n649 = call "ROB info data insert.vi"("error in (no error)"=w1198, "Data in"=w1199, "Hist cluster"=w1196) -> ("error out"=w1197:errorcluster)  [unwired: 8 in]
                    }
                    frame "Transm." {
                      n650 = call "Handle transmission status bytes.vi"("error in"=w1202, "Data in"=w1203, "All ROBs info cluster"=w1200) -> ("error out"=w1201:errorcluster)  [unwired: 8 in]
                    }
                    frame "Error/Success" {
                      n651 = call "Handle Error status bytes.vi"("error in (no error)"=w1204, "Data in"=w1206, "Hist cluster"=w1207) -> ("error out"=w1205:errorcluster)  [unwired: 8 in]
                    }
                  }
                }
              }
            }
          }
          frame "ResetCharts" {
            n652 = control-ref of="Bottom layer hit charts"() -> (w1213:refnum<vi>)
            n653 = control-ref of="Top layer hit charts"() -> (w1212:refnum<vi>)
            n654 = control-ref of="TDCStart time"() -> (w1209:refnum<vi>)
            n655 = call "ResetChartd.vi"("error in (no error)"=w1211, "reference"=w1209, "Bottom"=w1212, "Top"=w1213) -> ("error out"=w1210:errorcluster)  [unwired: 7 in]
          }
        }
      }
      frame Error {
        w1229 = "Stop" ("Single command")
        w1248 = "CommandQueue" ("name (unnamed)")
        n656 = property on="StopNotifier" class="TypRef (strict)"() -> (error out=w1245:errorcluster, "Value"=w1246:refnum<notifier>)  [unwired: 2 in, 1 out]
        n657 = property on="GPS serial port" class="VISAName"() -> (error out=w1215:errorcluster, "Value"=w1216:refnum<visa-resource-name>)  [unwired: 2 in, 1 out]
        n658 = property on="ROB serial port" class="VISAName"() -> (error out=w1240:errorcluster, "Value"=w1241:refnum<visa-resource-name>)  [unwired: 2 in, 1 out]
        n659 = property on="Master serial port" class="VISAName"() -> (error out=w1238:errorcluster, "Value"=w1239:refnum<visa-resource-name>)  [unwired: 2 in, 1 out]
        n660 = property on="Sniffer serial port" class="VISAName"() -> (error out=w1243:errorcluster, "Value"=w1242:refnum<visa-resource-name>)  [unwired: 2 in, 1 out]
        n661 = Obtain Queue(name (unnamed)=w1248, element data type=w1248) -> (queue out=w1251:refnum<queue>, error out=w1250:errorcluster)  [unwired: 3 in, 1 out]
        n662 = VISA Close(VISA resource name=w1241, error in (no error)=w1240) -> (error out=w1235:errorcluster)
        n663 = Send Notification(notification=TRUE, notifier=w1246, error in (no error)=w1245) -> (error out=w1237:errorcluster)  [unwired: 1 out]
        n664 = VISA Close(VISA resource name=w1239, error in (no error)=w1238) -> (error out=w1236:errorcluster)
        n665 = VISA Close(VISA resource name=w1242, error in (no error)=w1243) -> (error out=w1247:errorcluster)
        n666 = call "Close serial.vi"("error in (no error)"=w1215, "VISA name"=w1216) -> ("error out"=w1214:errorcluster)  [unwired: 9 in]
        n667 = Release Queue(queue=w1251, force destroy? (F)=TRUE, error in (no error)=w1250) -> (error out=w1217:errorcluster)  [unwired: 2 out]
        n668 = call "Append to command queue.vi"("Name (CommandQueue)"="CoincChara" ("Single command"), "Single command"=w1229) -> ("error out"=w1230:errorcluster)  [unwired: 9 in]
        n669 = call "Append to command queue.vi"("Name (CommandQueue)"="TCQ" ("Single command"), "Single command"=w1229) -> ("error out"=w1232:errorcluster)  [unwired: 9 in]
        n670 = call "Append to TDC command queue.vi"("Single command"=w1229) -> ("error out"=w1234:errorcluster)  [unwired: 10 in]
        n671 = Merge Errors(w1230, w1232, w1234, w1237, w1235, w1236, w1247, w1214, w1217, w1218) -> (w1222:errorcluster)
        n672 = global write "AllowTDCHitsRead.vi" "AllowTDCHitsRead"(FALSE ("AllowTDCHitsRead")) -> ()
        n673 = global write "Global AllowRead.vi" "Global allow TDC read"(FALSE ("AllowRead")) -> ()
        n674 = call <vilib>:"Stop Timed Structure.vi"("name"="autoreadtimer") -> ("error out"=w1223:errorcluster)  [unwired: 10 in]
        n675 = call <vilib>:"Stop Timed Structure.vi"("name"="hitratechecker") -> ("error out"=w1219:errorcluster)  [unwired: 10 in]
        n676 = call <vilib>:"Stop Timed Structure.vi"("name"="DayChecker") -> ("error out"=w1224:errorcluster)  [unwired: 10 in]
        n677 = Merge Errors(w1219, w1223, w1224, w1222) -> (w1221:errorcluster)
      }
    }
  }
  n678 = while {
    tunnel: w39 -> [w1276]
    shift-right: [w1274] -> w9
    shift-left: w2 -> [w1270]
    shift-right: [w1273] -> w12
    shift-left: "TDCManager" -> [w1271]
    stop <- w1265 stop-if-true
    n679 = Not A Number/Path/Refnum?(number/path/refnum=w1271) -> (NaN/Path/Refnum?=w1272:bool)
    n680 = Get Queue Status(queue=w1276, return elements? (F)=TRUE, error in (no error)=w1270) -> (queue out=w1280:refnum<queue>, error out=w1279:errorcluster, # elements in queue=w1281:i32, elements=→"TDC Command Queue":string[])  [unwired: 4 out]
    n681 = case shown="False" w1272 {
      tunnel: w1271 -> [w1286 w1287]
      tunnel: w1270 -> [w1285 w1288]
      tunnel: [w1284 w1288] -> w1268
      tunnel: [w1283 w1287] -> w1266
      frame False {
        n682 = call "Get State.vi"("error in"=w1285, "TDCManager"=w1286) -> ("error out"=w1284:errorcluster, "State"=→"Status":i32, "TDCManager"=w1283:T9)  [unwired: 6 in, 1 out]
      }
      frame True {
      }
    }
    n683 = case shown="0" w1281 {
      tunnel: ["Idle" ("element") w1448] -> w1275
      tunnel: w1280 -> [_ w1454]
      tunnel: w1279 -> [w1444 w1453]
      tunnel: [w1444 w1447] -> w1269
      frame 0 {
      }
      frame Default {
        n684 = Dequeue Element(queue=w1454, timeout in ms (-1)=10, error in (no error)=w1453) -> (element=w1452:string, timed out?=w1451:bool, error out=w1447:errorcluster)  [unwired: 1 out]
        n685 = Not(x=w1451) -> (.not. x?=w1450:bool)
        n686 = Select(t=w1452, s=w1450, f="TimeOut") -> (s? t:f=w1448:string)
      }
    }
    n687 = Merge Errors(w1268, w1269) -> (w1267:errorcluster)
    n688 = case shown="No Error" w1267 {
      selector: w1267 -> [w1293 w1428]
      tunnel: w1275 -> [w1294 _]
      tunnel: [w1292 w1424] -> w1274
      tunnel: [w1291 w1420] -> w1273
      tunnel: w1266 -> [w1290 w1425]
      tunnel: [w1289 TRUE] -> w1265
      frame No Error {
        n689 = case shown="\"TimeOut\"" w1294 {
          selector: w1294 -> [_ _ w1302 _ _ _ _ _ _ w1378 _ _ _]
          tunnel: w1293 -> [w1295 w1298 w1301 w1310 w1316 w1326 w1331 w1336 w1341 w1380 w1410 w1414 w1419]
          tunnel: [w1295 w1298 w1301 w1309 w1313 w1327 w1328 w1333 w1340 w1376 w1407 w1411 w1416] -> w1292
          tunnel: [w1296 w1299 w1300 w1307 w1312 w1322 w1329 w1334 w1339 w1374 w1408 w1412 w1417] -> w1291
          tunnel: w1290 -> [w1296 w1299 w1300 _ w1319 w1323 w1330 w1335 w1337 w1381 w1409 w1413 w1418]
          tunnel: [_ _ _ _ _ _ _ _ _ w1379 _ _ _] -> w1289
          frame "TimeOut" {
          }
          frame "Idle" {
            n690 = Wait (ms)(milliseconds to wait=u32 100) -> ()  [unwired: 1 out]
          }
          frame Default {
            n691 = Concatenate Strings(w1302, " is not valid command for TDC state machine." ("string")) -> (w1303:string)
            n692 = flat-sequence {
              tunnel: w1303 -> [w1305]
              frame #0 {
                n693 = call "Display Message to User3"("Message"=w1305) -> ()  [unwired: 9 in, 2 out]
              }
              frame #1 {
                n694 = Wait (ms)(milliseconds to wait=u32 200) -> ()  [unwired: 1 out]
              }
            }
          }
          frame "InitTDC" {
            n695 = call "Initiate.vi"("error in"=w1310, "Configuration filepath"="TDC Configuration filepath") -> ("error out"=w1309:errorcluster, "Success?"=w1308:bool, "TDCManager"=w1307:T9)  [unwired: 7 in]
            "Init success" <- w1308
            n696 = case shown="False" w1308 {
              frame False {
                n697 = call "Display Message to User4"() -> ()  [unwired: 10 in, 2 out]
              }
              frame True {
              }
            }
          }
          frame "LoadCfgFile" {
            n698 = property on="TDC Configuration filepath" class="Str"(error in=w1316) -> (error out=w1317:errorcluster, "Value"=w1318:string)  [unwired: 1 in, 1 out]
            n699 = call "Read Configuration File.vi"("error in (no error)"=w1317, "Configuration filepath"=w1318, "TDCManager"=w1319) -> ("error out"=w1315:errorcluster, "Success?"=w1314:bool, "TDCManager"=w1312:T9)  [unwired: 6 in]
            n700 = property on="Init success" class="Bool (strict)"(error in=w1315, "Value"=w1314) -> (error out=w1313:errorcluster)  [unwired: 1 in, 1 out]
            n701 = case shown="False" w1314 {
              frame False {
                n702 = call "Display Message to User5"() -> ()  [unwired: 10 in, 2 out]
              }
              frame True {
              }
            }
          }
          frame "ReadCfgFileAgain" {
            n703 = property on="TDC Configuration filepath" class="Str"(error in=w1326) -> (error out=w1325:errorcluster, "Value"=w1324:string)  [unwired: 1 in, 1 out]
            n704 = call "Read Configuration File.vi"("error in (no error)"=w1325, "Configuration filepath"=w1324, "TDCManager"=w1323) -> ("error out"=w1320:errorcluster, "Success?"=w1321:bool, "TDCManager"=w1322:T9)  [unwired: 6 in]
            n705 = property on="Init success" class="Bool (strict)"(error in=w1320, "Value"=w1321) -> (error out=w1327:errorcluster)  [unwired: 1 in, 1 out]
          }
          frame "Reconfigure" {
            n706 = call "Reconfigure.vi"("error in (no error)"=w1331, "TDCManager"=w1330) -> ("error out"=w1328:errorcluster, "TDCManager"=w1329:T9)  [unwired: 8 in]
          }
          frame "ReadCfgString" {
            n707 = call "Read Configuration String.vi"("error in (no error)"=w1336, "Config string"="TDC Config string", "TDCManager"=w1335) -> ("error out"=w1333:errorcluster, "TDCManager"=w1334:T9)  [unwired: 6 in, 1 out]
          }
          frame "StartTDC" {
            n708 = Not A Number/Path/Refnum?(number/path/refnum=w1337) -> (NaN/Path/Refnum?=w1338:bool)
            n709 = case shown="False" w1338 {
              tunnel: w1341 -> [w1342 w1369]
              tunnel: [w1347 w1368] -> w1340
              tunnel: [w1346 w1373] -> w1339
              tunnel: w1337 -> [w1345 w1373]
              frame False {
                n710 = property on="Status" class="Ring (strict)"(error in=w1342) -> (error out=w1343:errorcluster, "Value"=w1344:u16)  [unwired: 1 in, 1 out]
                n711 = case shown="Default" w1344 {
                  tunnel: w1343 -> [w1348 w1356]
                  tunnel: [w1349 w1355] -> w1347
                  tunnel: [w1351 w1353] -> w1346
                  tunnel: w1345 -> [w1351 w1354]
                  frame 9 {
                    n712 = call "Append to TDC command queue.vi"("error in (no error)"=w1348, "Single command"="LoadCfgFile") -> ("error out"=w1349:errorcluster)  [unwired: 9 in]
                  }
                  frame Default {
                    n713 = flat-sequence {
                      tunnel: w1356 -> [w1362]
                      tunnel: [w1359] -> w1355
                      tunnel: w1354 -> [w1361]
                      tunnel: [w1360] -> w1352
                      tunnel: [w1367] -> w1353
                      tunnel: w1352 -> [w1367]
                      frame #0 {
                        n714 = call "Start.vi"("error in (no error)"=w1362, "TDCManager"=w1361) -> ("error out"=w1359:errorcluster, "Added time"=→"Added time":u64, "TDCManager"=w1360:T9)  [unwired: 6 in, 1 out]
                        n715 = local write "TDCManager"(w1360) -> ()
                        n716 = call "TDCTime.vi"("Enum"=enum16{"Get", "Init"}."Init") -> ()  [unwired: 1 out]
                      }
                      frame #1 {
                        n717 = property on="Fast read" class="Bool (strict)"() -> ("Value"=w1365:bool)  [unwired: 2 in, 2 out]
                        n718 = Get Date/Time In Seconds() -> (seconds since 1Jan1904=→"TDCStart time":timestamp)
                        n719 = global write "Global AllowRead.vi" "Global allow TDC read"(TRUE ("AllowRead")) -> ()
                        n720 = Not(x=w1365) -> (.not. x?=w1364:bool)
                        n721 = global write "AllowTDCHitsRead.vi" "AllowTDCHitsRead"(w1364) -> ()
                        n722 = global write "AllowTDCFastRead.vi" "AllowTDCFastRead"(w1365) -> ()
                      }
                    }
                  }
                }
              }
              frame True {
                n723 = call "Append to TDC command queue.vi"("error in (no error)"=w1369, "Single command"="InitTDC") -> ("error out"=w1372:errorcluster)  [unwired: 9 in]
                n724 = call "Append to TDC command queue.vi"("error in (no error)"=w1372, "Single command"="StartTDC") -> ("error out"=w1368:errorcluster)  [unwired: 9 in]
              }
            }
          }
          frame "Stop", "StopTDC" {
            n725 = Not A Number/Path/Refnum?(number/path/refnum=w1381) -> (NaN/Path/Refnum?=w1382:bool)
            n726 = case shown="False" w1382 {
              tunnel: w1381 -> [w1395 w1406]
              tunnel: [w1397 w1405] -> w1377
              tunnel: w1380 -> [w1394 w1405]
              tunnel: [w1396 w1406] -> w1375
              frame False {
                n727 = flat-sequence {
                  tunnel: w1394 -> [w1399]
                  tunnel: w1395 -> [w1400]
                  tunnel: [w1400] -> w1393
                  tunnel: [w1399] -> w1392
                  tunnel: [w1404] -> w1397
                  tunnel: [w1403] -> w1396
                  tunnel: w1393 -> [w1402]
                  tunnel: w1392 -> [w1401]
                  frame #0 {
                    w1398 = FALSE ("AllowRead")
                    n728 = global write "AllowTDCHitsRead.vi" "AllowTDCHitsRead"(w1398) -> ()
                    n729 = global write "AllowTDCFastRead.vi" "AllowTDCFastRead"(w1398) -> ()
                    n730 = global write "Global AllowRead.vi" "Global allow TDC read"(w1398) -> ()
                  }
                  frame #1 {
                    n731 = call "Stop.vi"("error in (no error)"=w1401, "TDCManager"=w1402) -> ("error out"=w1404:errorcluster, "TDCManager"=w1403:T9)  [unwired: 8 in]
                  }
                }
              }
              frame True {
              }
            }
            n732 = case shown="\"Stop\"" w1378 {
              tunnel: [FALSE TRUE] -> w1379
              tunnel: w1377 -> [w1383 w1387]
              tunnel: [w1383 w1390] -> w1376
              tunnel: w1375 -> [w1384 w1389]
              tunnel: [w1384 w1388] -> w1374
              frame "StopTDC", Default {
              }
              frame "Stop" {
                n733 = call "Clean Up.vi"("error in (no error)"=w1387, "TDCManager"=w1389) -> ("error out"=w1386:errorcluster, "TDCManager out"=w1388:T9)  [unwired: 8 in]
                n734 = Merge Errors(w1386) -> (w1390:errorcluster)
              }
            }
          }
          frame "PauseTDC" {
            n735 = call "Pause.vi"("error in (no error)"=w1410, "TDCManager"=w1409) -> ("error out"=w1407:errorcluster, "TDCManager"=w1408:T9)  [unwired: 8 in]
          }
          frame "ContinueTDC" {
            n736 = call "Continue.vi"("error in (no error)"=w1414, "TDCManager"=w1413) -> ("error out"=w1411:errorcluster, "TDCManager"=w1412:T9)  [unwired: 8 in]
          }
          frame "GetParams" {
            n737 = call "Get Parameter Names.vi"("error in (no error)"=w1419, "TDCManager"=w1418) -> ("error out"=w1416:errorcluster, "Parameter Names"=→"Set Parameter Names":string[], "TDCManager"=w1417:T9)  [unwired: 7 in]
          }
        }
      }
      frame Error {
        n738 = Not A Number/Path/Refnum?(number/path/refnum=w1425) -> (NaN/Path/Refnum?=w1426:bool)
        n739 = case shown="False" w1426 {
          tunnel: w1425 -> [w1433 w1443]
          tunnel: [w1434 _] -> w1422
          tunnel: [w1432 _] -> w1421
          tunnel: [w1431 w1443] -> w1420
          frame False {
            n740 = flat-sequence {
              tunnel: w1433 -> [w1437]
              tunnel: [w1437] -> w1430
              tunnel: [w1442] -> w1434
              tunnel: [w1439] -> w1432
              tunnel: [w1438] -> w1431
              tunnel: w1430 -> [w1440]
              frame #0 {
                n741 = global write "AllowTDCHitsRead.vi" "AllowTDCHitsRead"(FALSE ("AllowTDCHitsRead")) -> ()
                n742 = global write "Global AllowRead.vi" "Global allow TDC read"(FALSE ("AllowRead")) -> ()
              }
              frame #1 {
                n743 = call "Stop.vi"("TDCManager"=w1440) -> ("error out"=w1439:errorcluster, "TDCManager"=w1441:T9)  [unwired: 9 in]
                n744 = call "Clean Up.vi"("TDCManager"=w1441) -> ("error out"=w1442:errorcluster, "TDCManager out"=w1438:T9)  [unwired: 9 in]
              }
            }
          }
          frame True {
          }
        }
        n745 = call "Append to command queue.vi"("Single command"="Stop") -> ("error out"=w1427:errorcluster)  [unwired: 10 in]
        n746 = Merge Errors(w1422, w1421, w1427, w1428) -> (w1424:errorcluster)
      }
    }
  }
  n747 = flat-sequence {
    tunnel: w2 -> [w1456]
    tunnel: [w1455] -> w1
    tunnel: [w1484] -> w41
    tunnel: w1 -> [w1460]
    frame #0 {
      n748 = while {
        tunnel: [w1459] -> w1455
        tunnel: w1456 -> [w1459]
        stop <- w1458 stop-if-true
        n749 = local read "Initiate finished"() -> (w1458:bool)
        n750 = Wait (ms)(milliseconds to wait=u32 10) -> ()  [unwired: 1 out]
      }
    }
    frame #1 {
      n751 = local read "hit charts refnum cluster"() -> (w1461:T12)
      n752 = control-ref of="Coinc stats time"() -> (w1471:refnum<vi>)
      n753 = control-ref of="Added time"() -> (w1470:refnum<vi>)
      n754 = control-ref of="Histograms cluster"() -> (w1473:refnum<vi>)
      n755 = control-ref of="Coinc stats table"() -> (w1472:refnum<vi>)
      n756 = call "HandleCoincidenceData.vi"("Added time"=w1470, "Seconds indicator"=w1471, "hit charts refnum cluster"=w1461, "error in (no error)"=w1460, "coinc table"=w1472, "Seconds between updates"=1, "Cluster"=w1473) -> ("error out"=w1475:errorcluster)  [unwired: 4 in]
      n757 = Unbundle By Name(w1461) -> ("Hit charts bottom"=w1463:T11, "Hit charts top"=w1462:T11)
      n758 = control-ref of="Daily datafile reference"() -> (w1483:refnum<vi>)
      n759 = control-ref of="ROB Info cluster"() -> (w1482:refnum<vi>)
      n760 = control-ref of="Run ID"() -> (w1481:refnum<vi>)
      n761 = control-ref of="Hit rate save granularity in minutes"() -> (w1467:refnum<vi>)
      n762 = control-ref of="ROB information save granularity in minutes"() -> (w1480:refnum<vi>)
      n763 = control-ref of="GPS information save granularity in minutes"() -> (w1469:refnum<vi>)
      n764 = Bundle(cluster=T30 {"Hit charts bottom"=refnum, "Hit charts top"=refnum, "Hitrate save granularity in minutes"=refnum} ("Hitrate save info"), "Hit charts bottom"=w1463, "Hit charts top"=w1462, "Hitrate save granularity in minutes"=w1467) -> (w1466:T30)
      n765 = call "Save CRT data to file.vi"("GPS data granularity (minutes)"=w1469, "Hitrate save info"=w1466, "ROB data granularity (minutes)"=w1480, "error in"=w1460, "Run ID"=w1481, "ROB Info cluster"=w1482, "HDF5 data file"=w1483) -> ("error out"=w1476:errorcluster)  [unwired: 4 in]
      n766 = control-ref of="Coincidences analysis overload"() -> (w1477:refnum<vi>)
      n767 = call "Layercoincidence.vi"("Coincidence result queue overflow ref"=w1477, "error in (no error)"=w1460, "Type"=T31."TopLayer") -> ("error out"=w1464:errorcluster)  [unwired: 8 in]
      n768 = call "Layercoincidence.vi"("Coincidence result queue overflow ref"=w1477, "error in (no error)"=w1460, "Type"=T31."BottomLayer") -> ("error out"=w1465:errorcluster)  [unwired: 8 in]
      n769 = Merge Errors(w1465, w1464, w1476, w1475) -> (w1484:errorcluster)
    }
  }
  n770 = node-c288(w18) -> ()  [unwired: 1 out]
  n771 = node-c288(w30) -> ()  [unwired: 1 out]
  n772 = node-c288(i64 10000 ("Period"), "DayChecker" ("Source Name")) -> (w23:T15)  [unwired: 3 in]
  n773 = timed-loop {
    timing: w23 -> [_]
    timing-out: [_] -> w22
    i -> [w1486]
    stop <- _ stop-if-true
    # "Switch savefiles if a new day has been entered."
    n774 = node-c288() -> ()  [unwired: 1 in, 1 out]
    n775 = global read "take CRT data.vi" "Save CRT data"() -> (w1485:bool)
    n776 = case shown="True" w1485 {
      tunnel: w1486 -> [_ w1487]
      frame False {
      }
      frame True {
        n777 = flat-sequence {
          tunnel: [w1489] -> w1488
          tunnel: w1488 -> [w1492]
          tunnel: w1487 -> [_]
          frame #0 {
            n778 = local read "Current day"() -> (w1489:i32)
          }
          frame #1 {
            n779 = Get Date/Time In Seconds() -> (seconds since 1Jan1904=w1495:timestamp)
            n780 = Format Date/Time String(time format string (%c)="%d", seconds (now)=w1495) -> (date/time string=w1493:string)  [unwired: 1 in]
            n781 = Decimal String To Number(string=w1493) -> (number=w1490:i32)  [unwired: 2 in, 1 out]
            "Current day" <- w1490
            n782 = Equal?(x=w1490, y=w1492) -> (x = y?=w1491:bool)
            n783 = case shown="False" w1491 {
              frame False {
                n784 = call "Append to command queue.vi"("Single command"="SwitchFiles") -> ()  [unwired: 10 in, 1 out]
              }
              frame True {
              }
            }
          }
        }
      }
    }
    n785 = node-c288() -> ()  [unwired: 1 in, 1 out]
  }
  n786 = Close Reference(reference=w12) -> (error out=w10:errorcluster)  [unwired: 1 in]
  n787 = Merge Errors(w10, w9) -> (w16:errorcluster)
  n788 = Merge Errors(w48, w41, w16) -> (w43:errorcluster)
  n789 = flat-sequence {
    tunnel: w43 -> [w1521]
    tunnel: [w1520] -> w34
    tunnel: [w1588] -> w42
    tunnel: w34 -> [w1589]
    frame #0 {
      # "Here we stop all asynchronously launched VIs and collect their errors."
      n790 = local read "Trig chara refnum"() -> (w1509:refnum<vi>)
      n791 = local read "TDCFastRead Refnum"() -> (w1556:refnum<vi>)
      n792 = local read "charactirzator refnum"() -> (w1499:refnum<vi>)
      n793 = local read "Event display Refnum"() -> (w1506:refnum<vi>)
      n794 = local read "MasterSerial Refnum"() -> (w1528:refnum<vi>)
      n795 = local read "SnifferSerial Refnum"() -> (w1529:refnum<vi>)
      n796 = local read "Master command sender refnum"() -> (w1517:refnum<vi>)
      n797 = local read "ROBSerial Refnum"() -> (w1530:refnum<vi>)
      n798 = local read "TDCRead Refnum"() -> (w1555:refnum<vi>)
      n799 = local read "GPSSerial Refnum"() -> (w1501:refnum<vi>)
      n800 = local read "Sorter Refnum"() -> (w1557:refnum<vi>)
      n801 = Not A Number/Path/Refnum?(number/path/refnum=w1506) -> (NaN/Path/Refnum?=w1507:bool)
      n802 = Not A Number/Path/Refnum?(number/path/refnum=w1509) -> (NaN/Path/Refnum?=w1510:bool)
      n803 = Not A Number/Path/Refnum?(number/path/refnum=w1499) -> (NaN/Path/Refnum?=w1508:bool)
      n804 = call-by-ref "Wait On Asynchronous Call"(reference=w1557) -> (reference out=w1552:refnum<vi>, error out=w1554:errorcluster, 0:"error out"=w1553:errorcluster)  [unwired: 12 in]
      n805 = call-by-ref "Wait On Asynchronous Call"(reference=w1556) -> (reference out=w1547:refnum<vi>, error out=w1549:errorcluster, 0:"error out"=w1548:errorcluster)  [unwired: 12 in]
      n806 = call-by-ref "Wait On Asynchronous Call"(reference=w1555) -> (reference out=w1545:refnum<vi>, error out=w1544:errorcluster, 0:"error out"=w1543:errorcluster)  [unwired: 12 in]
      n807 = call-by-ref "Wait On Asynchronous Call"(reference=w1530) -> (reference out=w1533:refnum<vi>, error out=w1531:errorcluster, 0:"error out"=w1532:errorcluster)  [unwired: 12 in]
      n808 = call-by-ref "Wait On Asynchronous Call"(reference=w1529) -> (reference out=w1538:refnum<vi>, error out=w1536:errorcluster, 0:"error out"=w1537:errorcluster)  [unwired: 12 in]
      n809 = case shown="False" w1510 {
        tunnel: [w1571 _] -> w1512
        tunnel: w1509 -> [w1570 _]
        frame False {
          n810 = call-by-ref "Wait On Asynchronous Call"(reference=w1570) -> (reference out=w1575:refnum<vi>, error out=w1573:errorcluster, "Error out"=w1572:errorcluster)  [unwired: 12 in]
          n811 = Close Reference(reference=w1575) -> (error out=w1574:errorcluster)  [unwired: 1 in]
          n812 = Merge Errors(w1574, w1573, w1572) -> (w1571:errorcluster)
        }
        frame True {
        }
      }
      n813 = call-by-ref "Wait On Asynchronous Call"(reference=w1528) -> (reference out=w1540:refnum<vi>, error out=w1541:errorcluster, 0:"error out"=w1542:errorcluster)  [unwired: 12 in]
      n814 = call-by-ref "Wait On Asynchronous Call"(reference=w1517) -> (reference out=w1514:refnum<vi>, error out=w1518:errorcluster, 0:"error out"=w1516:errorcluster)  [unwired: 12 in]
      n815 = case shown="False" w1507 {
        tunnel: [w1560 _] -> w1513
        tunnel: w1506 -> [w1558 _]
        frame False {
          n816 = call-by-ref "Wait On Asynchronous Call"(reference=w1558) -> (reference out=w1559:refnum<vi>, error out=w1562:errorcluster, 0:"error out"=w1563:errorcluster)  [unwired: 12 in]
          n817 = Close Reference(reference=w1559) -> (error out=w1561:errorcluster)  [unwired: 1 in]
          n818 = Merge Errors(w1561, w1562, w1563) -> (w1560:errorcluster)
        }
        frame True {
        }
      }
      n819 = case shown="False" w1508 {
        tunnel: w1499 -> [w1565 _]
        tunnel: [w1564 _] -> w1511
        frame False {
          n820 = call-by-ref "Wait On Asynchronous Call"(reference=w1565) -> (reference out=w1566:refnum<vi>, error out=w1568:errorcluster, "Error out"=w1569:errorcluster)  [unwired: 12 in]
          n821 = Close Reference(reference=w1566) -> (error out=w1567:errorcluster)  [unwired: 1 in]
          n822 = Merge Errors(w1567, w1568, w1569) -> (w1564:errorcluster)
        }
        frame True {
        }
      }
      n823 = call-by-ref "Wait On Asynchronous Call"(reference=w1501) -> (reference out=w1502:refnum<vi>, error out=w1504:errorcluster, 0:"error out"=w1503:errorcluster)  [unwired: 12 in]
      n824 = Close Reference(reference=w1547) -> (error out=w1550:errorcluster)  [unwired: 1 in]
      n825 = Close Reference(reference=w1552) -> (error out=w1551:errorcluster)  [unwired: 1 in]
      n826 = Close Reference(reference=w1545) -> (error out=w1546:errorcluster)  [unwired: 1 in]
      n827 = Close Reference(reference=w1538) -> (error out=w1535:errorcluster)  [unwired: 1 in]
      n828 = Close Reference(reference=w1533) -> (error out=w1534:errorcluster)  [unwired: 1 in]
      n829 = Close Reference(reference=w1540) -> (error out=w1539:errorcluster)  [unwired: 1 in]
      n830 = Close Reference(reference=w1514) -> (error out=w1519:errorcluster)  [unwired: 1 in]
      n831 = Close Reference(reference=w1502) -> (error out=w1505:errorcluster)  [unwired: 1 in]
      n832 = Merge Errors(w1550, w1549, w1548) -> (w1526:errorcluster)
      n833 = Merge Errors(w1551, w1554, w1553) -> (w1527:errorcluster)
      n834 = Merge Errors(w1546, w1544, w1543) -> (w1525:errorcluster)
      n835 = Merge Errors(w1535, w1536, w1537) -> (w1523:errorcluster)
      n836 = Merge Errors(w1534, w1531, w1532) -> (w1524:errorcluster)
      n837 = Merge Errors(w1539, w1541, w1542) -> (w1522:errorcluster)
      n838 = Merge Errors(w1519, w1518, w1516) -> (w1515:errorcluster)
      n839 = Merge Errors(w1505, w1504, w1503) -> (w1500:errorcluster)
      n840 = Merge Errors(w1521, w1527, w1526, w1525, w1524, w1523, w1522, w1515, w1513, w1512, w1511, w1500) -> (w1520:errorcluster)
    }
    frame #1 {
      # "Release queues and notifiers."
      n841 = property on="TDCHitsQueue" class="TypRef (strict)"() -> (error out=w1586:errorcluster, "Value"=w1587:refnum<queue>)  [unwired: 2 in, 1 out]
      n842 = property on="MasterCmdQueue" class="TypRef (strict)"() -> (error out=w1581:errorcluster, "Value"=w1582:refnum<queue>)  [unwired: 2 in, 1 out]
      n843 = property on="StopNotifier" class="TypRef (strict)"() -> (error out=w1592:errorcluster, "Value"=w1593:refnum<notifier>)  [unwired: 2 in, 1 out]
      n844 = property on="GpsDataQueue" class="TypRef (strict)"() -> (error out=w1577:errorcluster, "Value"=w1578:refnum<queue>)  [unwired: 2 in, 1 out]
      n845 = Release Notifier(notifier=w1593, force destroy? (F)=FALSE, error in (no error)=w1592) -> (error out=w1590:errorcluster)  [unwired: 2 out]
      n846 = Release Queue(queue=w1587, force destroy? (F)=TRUE, error in (no error)=w1586) -> (error out=w1584:errorcluster)  [unwired: 2 out]
      n847 = Release Queue(queue=w1582, force destroy? (F)=TRUE, error in (no error)=w1581) -> (error out=w1580:errorcluster)  [unwired: 2 out]
      n848 = Release Queue(queue=w1578, force destroy? (F)=TRUE, error in (no error)=w1577) -> (error out=w1576:errorcluster)  [unwired: 2 out]
      n849 = Merge Errors(w1589, w1590, w1584, w1580, w1576) -> (w1588:errorcluster)
    }
  }
  n850 = node-c288(w22) -> ()  [unwired: 1 out]
  "error out" <- w42
